vi "EnFlo_Lab_Temp_Control.vi"(0 "Current Time":dbl) -> ()   [LabVIEW 2022 SP3]
uses:
  Anemometry/Anemometry Sub Vis/Globals/EnFlo_Tunnel_Global.vi
  <vilib>/Analysis/NI_AALPro.lvlib
panel:
  in  "Don't Use Fan Heaters":bool
  in  "Don't Use Exit Heaters":bool
  out "At Maximum Heating":bool
  out "At Maximum Cooling":bool
  out "Back End Chiller Cooling Max":bool
  out "Back End Chiller Heating Max":bool
  out "Exit Heaters Max":bool
  out "Fan Heater Max":bool
  out "Volcano Max":bool
  out "Vent Max":bool
  out "Back End Chiller Cooling (kW)":dbl
  out "Ventilation Cooling (kW)":dbl
  out "Volcano Cooling (kW)":dbl
  out "Heat input to lab from Hot Pipework (kW)":dbl
  out "EnFlo_Lab Shut Down":bool
  in  "Paint Spraying by South West Fan":bool
  in  "Lab Fan heaters in kW":dbl=3.0
  in  "Don't Use Volcano":bool
  in  "Don't Use Ventilation":bool
  in  "Volcano Cooling kW":dbl=15.0
  in  "Manual Ventilation %":dbl=50.0
  in  "Lab Ventilation % during Ozone Exp":dbl
  in  "Ozone Averaging time (mins)":dbl=2.0
  in  "O3 Generator Control":T1={"Gen Output 0, Imin (mA)"=4.0, "USB3102 Number"=0.0, "DO O3 Gen Power"=0, "AO O3 Gen"=0, "O3 Gen Limit, Imax (mA)"=10.0, "Smoothing factor 0<1"=0.14} {"Smoothing factor 0<1" min=0.0 max=1.0 step=0.01; "AO O3 Gen" min=0 max=2 step=1; "DO O3 Gen Power" min=0 max=7 step=1}
  out "Ventilation Cooling limit in kW":dbl
  in  "Kp Ventilation":dbl=1.8
  out "Lab Reference Temperature":dbl
  out "Derivative Short":dbl(graph)
  in  "Kd Long":dbl=6000.0 format="%.2f"
  in  "Derivative Short History":i32=9
  in  "Exit Heater Power in kW":dbl=12.0
  out "Error":dbl(graph)
  out "Derivative Long":dbl(graph)
  out "integral":dbl(graph)
  out "Proportional":dbl(graph)
  out "Integral Term":dbl
  out "Derivative Term":dbl
  out "Proportional Term":dbl
  out "Cooling from Tunnel Exit Duct kW":dbl
  out "Exit Heater Dem Power %":dbl
  in  "Ki":dbl=0.013 format="%.3f"
  in  "Kp":dbl=3.0 format="%.2f"
  in  "Kd short":dbl=500.0 format="%.2f"
  in  "Derivative Long History":i32=35
  out "EnFlo Lab:labstrat1:Av Temp":dbl
  out "EnFlo_Tunnel:Exit Duct:Dem Temp":dbl
  out "Reduction in air temp from ambient":dbl
  out "Heat Extraction Value in kW":dbl
  out "EnFlo Lab:Desired:Air Temp":dbl
  out "Temperature Error":dbl
  # "USB 3102 Channel Numbers"
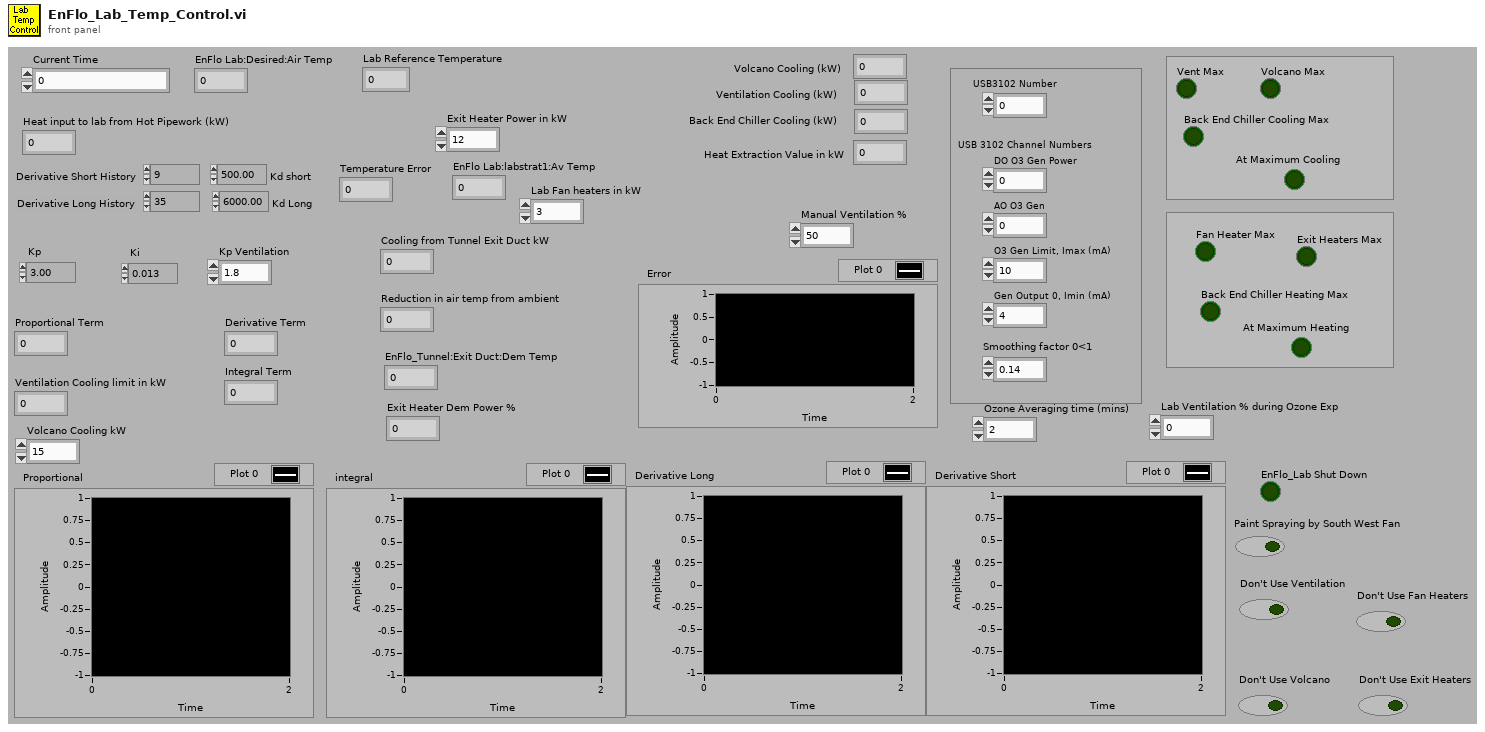
[diagram p1: front panel]
types:
  T1 = cluster{"Gen Output 0, Imin (mA)":sgl, "USB3102 Number":dbl, "DO O3 Gen Power":i32, "AO O3 Gen":i16, "O3 Gen Limit, Imax (mA)":dbl, "Smoothing factor 0<1":dbl}
  T2 = cluster{"second":i32, "minute":i32, "hour":i32, "day of month":i32, "month":i32, "year":i32, "day of week":i32, "day of year":i32, "is DST":i32}
  T3 = enum16{"Append to Global", "Read Global then Clear"}
  T4 = typedef "Ch_description_ADAM.ctl" = cluster{"Ch Name":string, "Type":T5, "Function":T6, "Ch State":T7, "Calibration type":T8, "A":dbl, "B":dbl, "C":dbl, "D":dbl, "Comments":string, "Address":T9, "String":string, "Duty":u16}
  T5 = typedef "Module_type_ADAM.ctl" = string
  T6 = typedef "Function_ADAM.ctl" = enum16{"Analogue Input", "Digital Input", "Event counter", "Event rate", "Analogue Output", "Digital Output", "Relay Output"}
  T7 = typedef "Channel_State.ctl" = enum16{"On", "Off", "Always On", "Always Off"}
  T8 = typedef "Calib_type_ADAM.ctl" = string
  T9 = typedef "Address.ctl" = cluster{"Main":i32, "Ch.":i32, "Sub":i32, "Port Name":string}
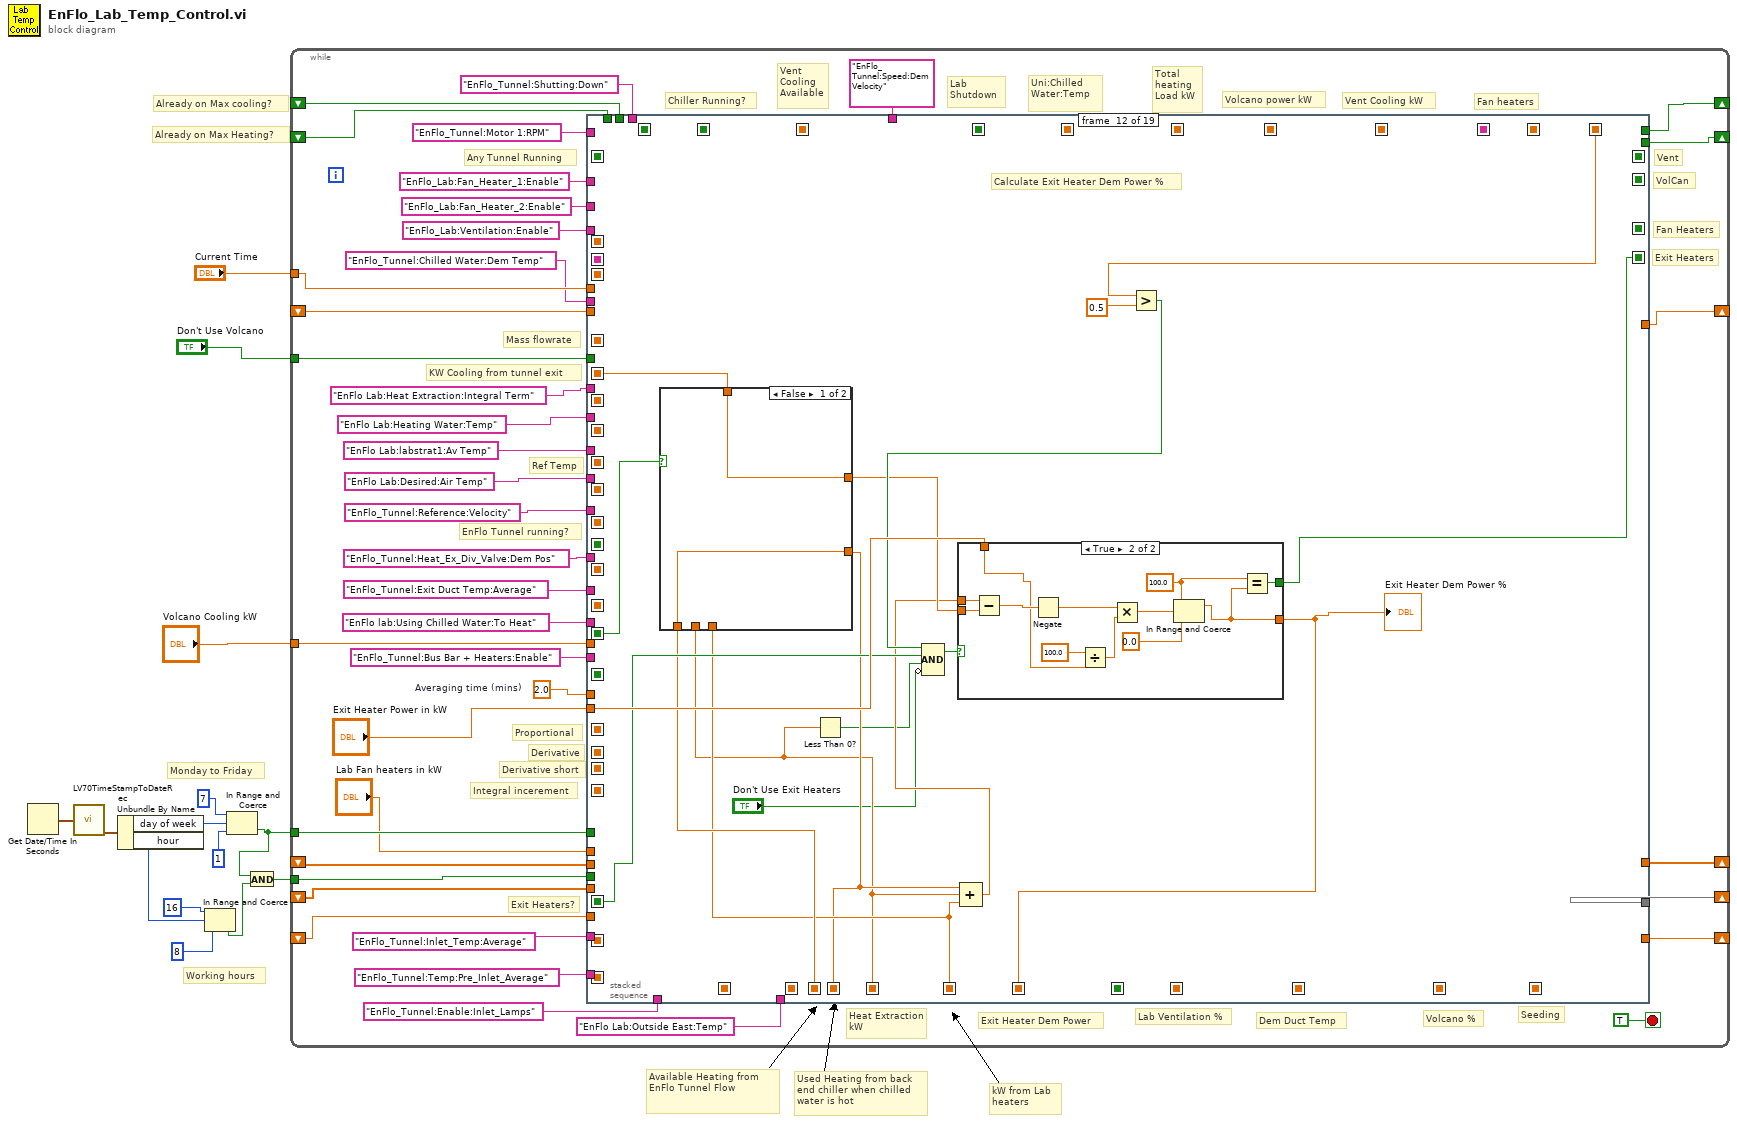
[diagram p0: block diagram]
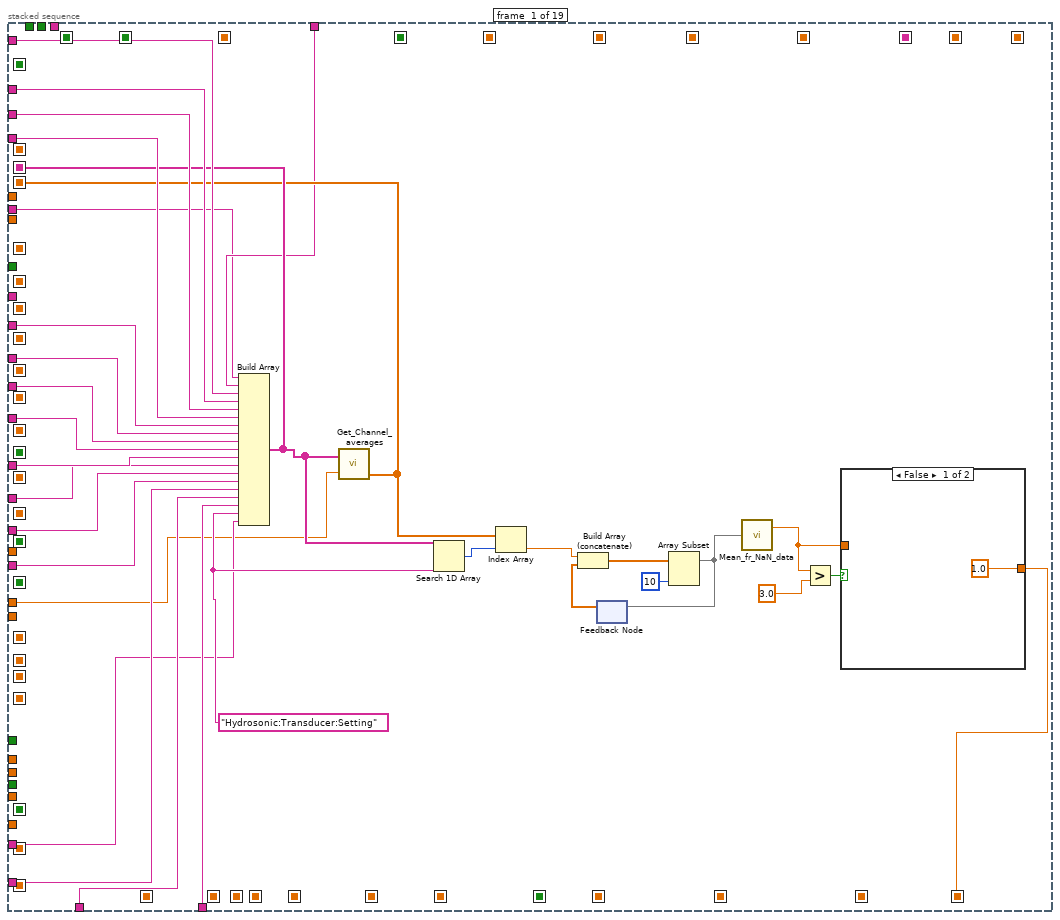
[diagram p2: hidden frame]
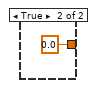
[diagram p3: hidden frame]
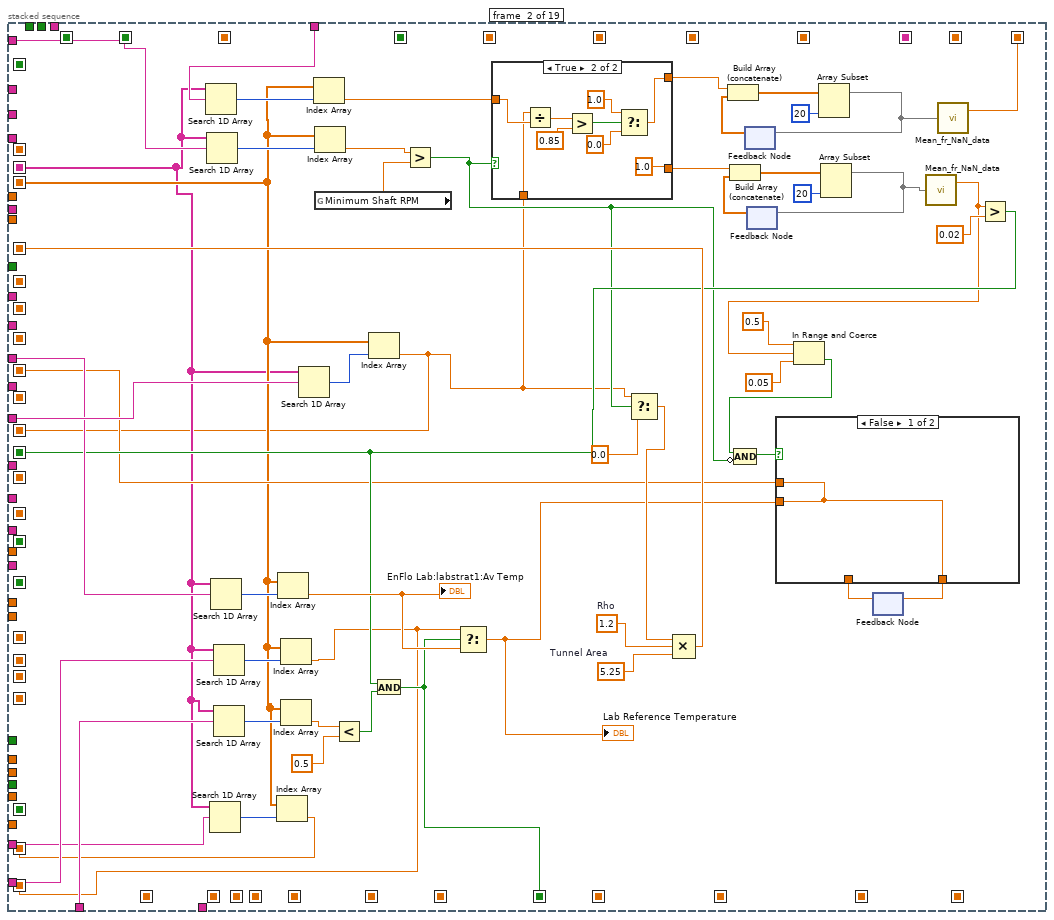
[diagram p4: hidden frame]
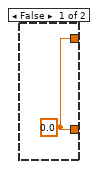
[diagram p5: hidden frame]
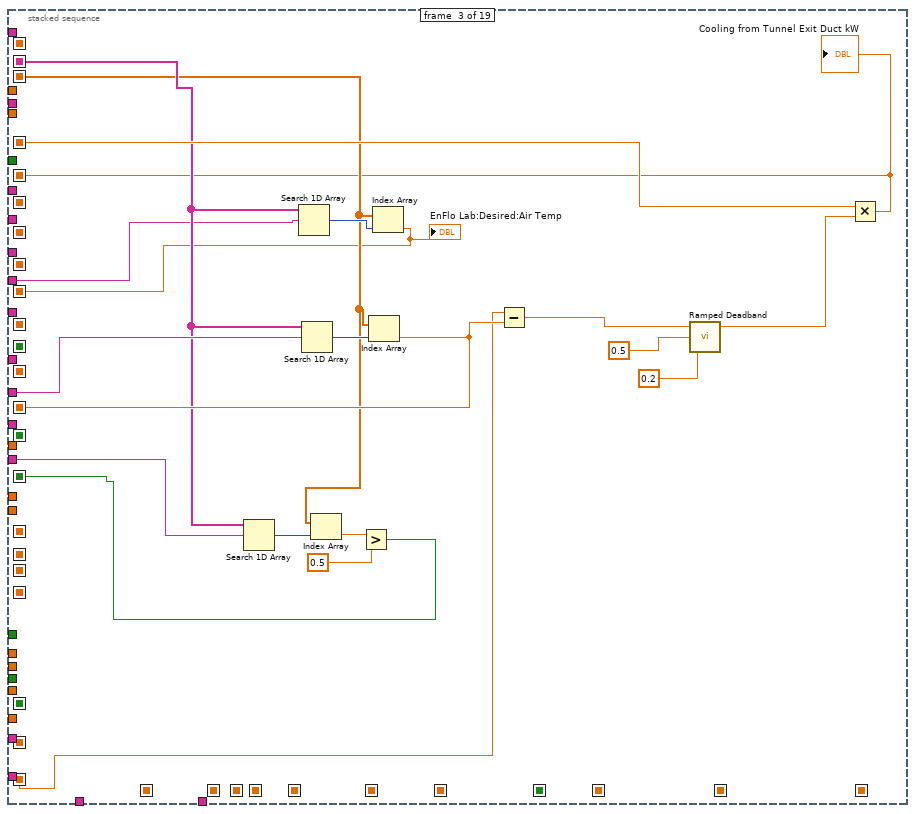
[diagram p7: hidden frame]
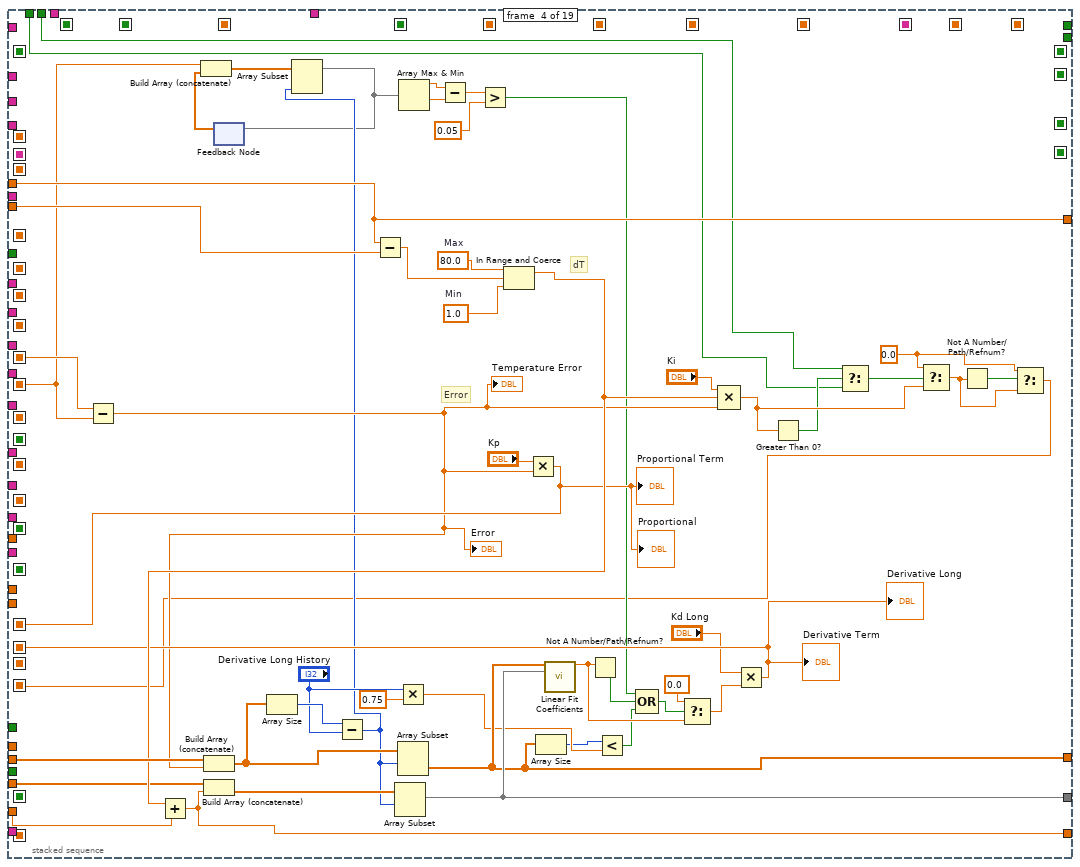
[diagram p8: hidden frame]
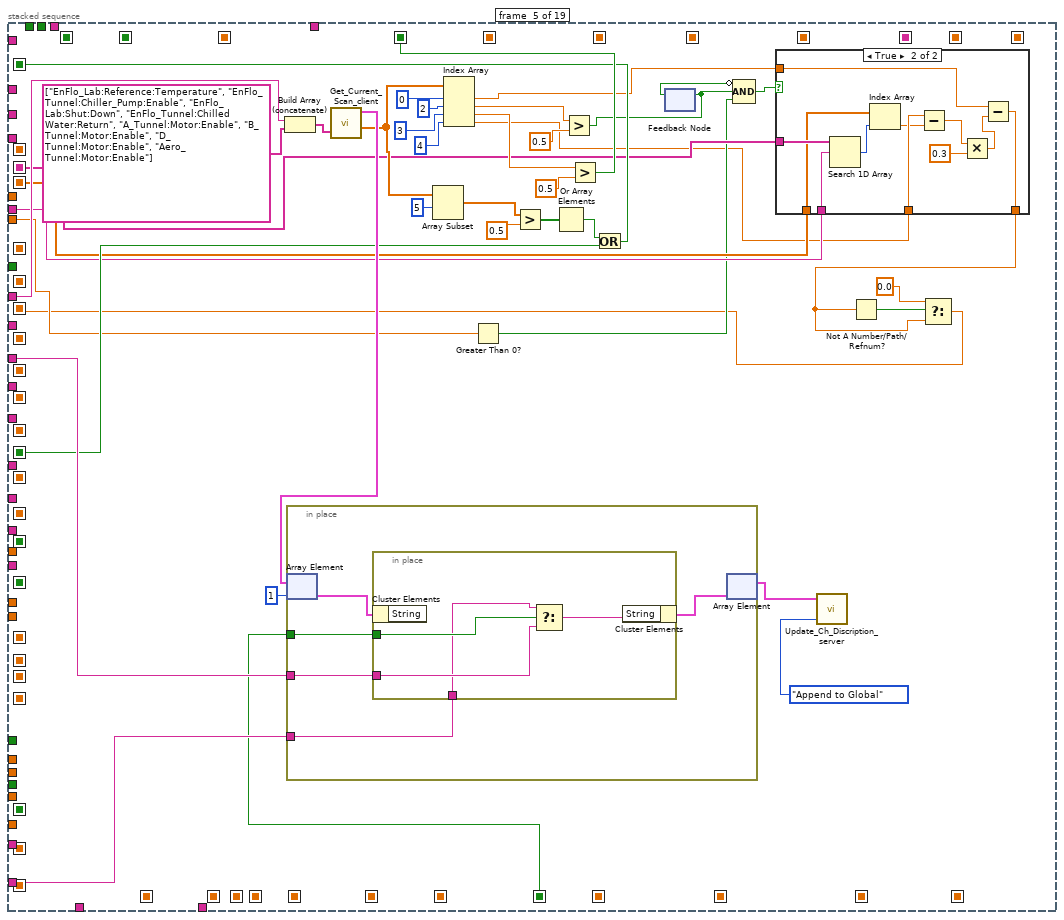
[diagram p9: hidden frame]
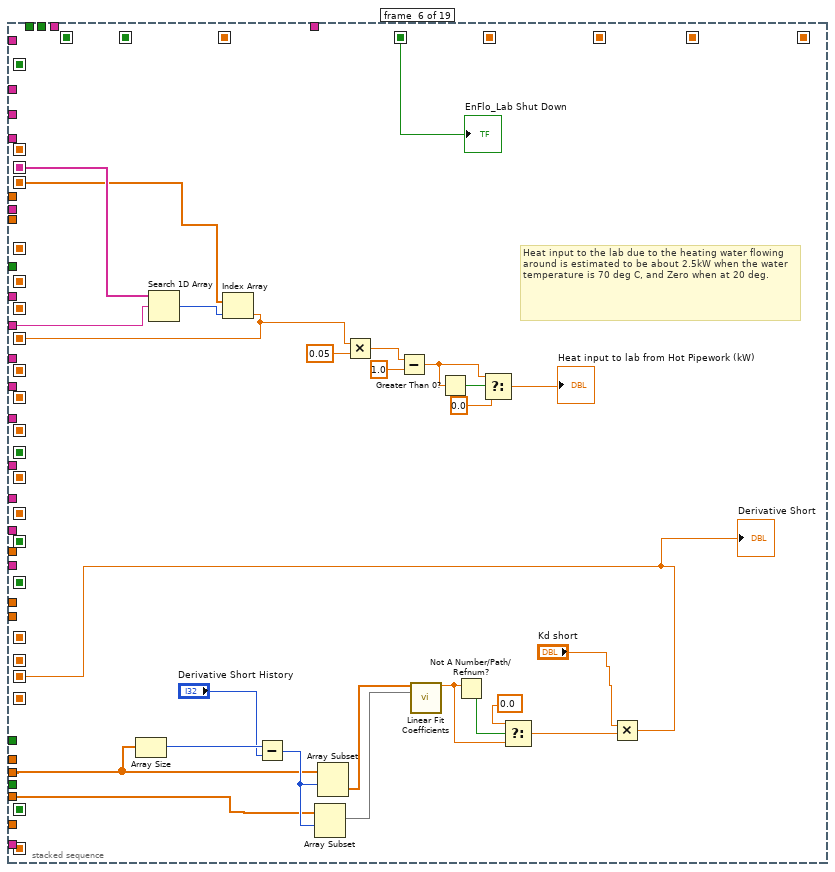
[diagram p11: hidden frame]
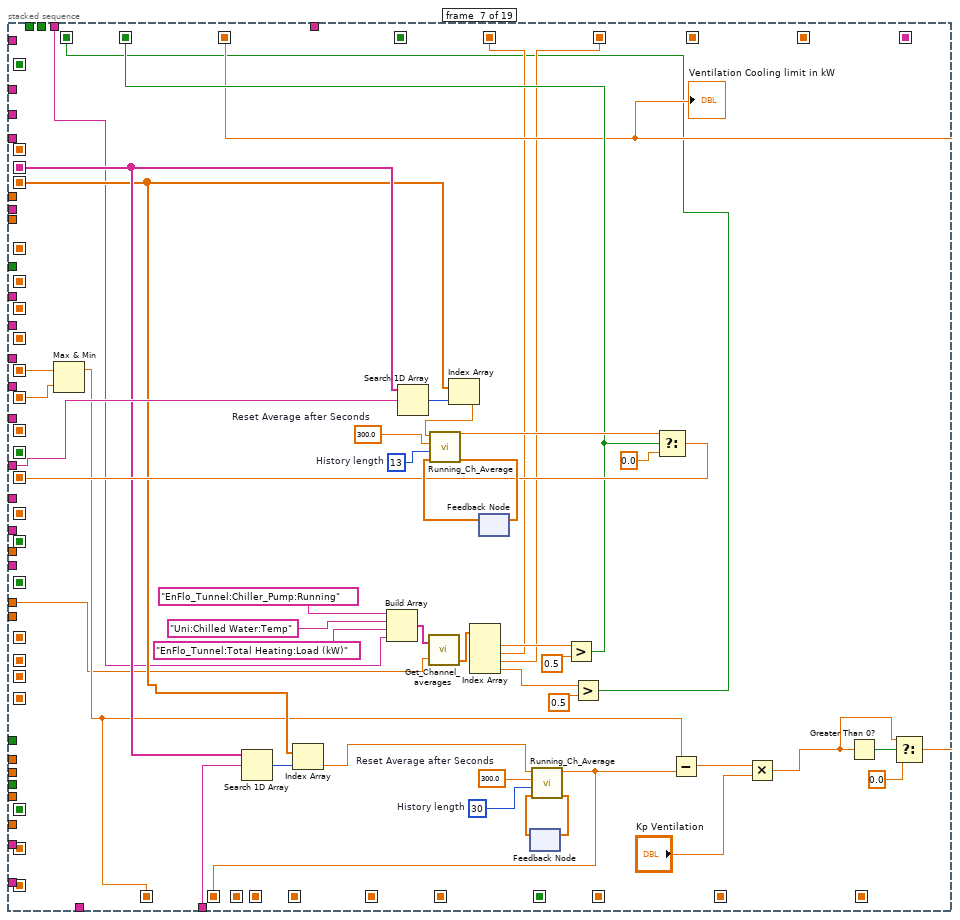
[diagram p12: hidden frame]
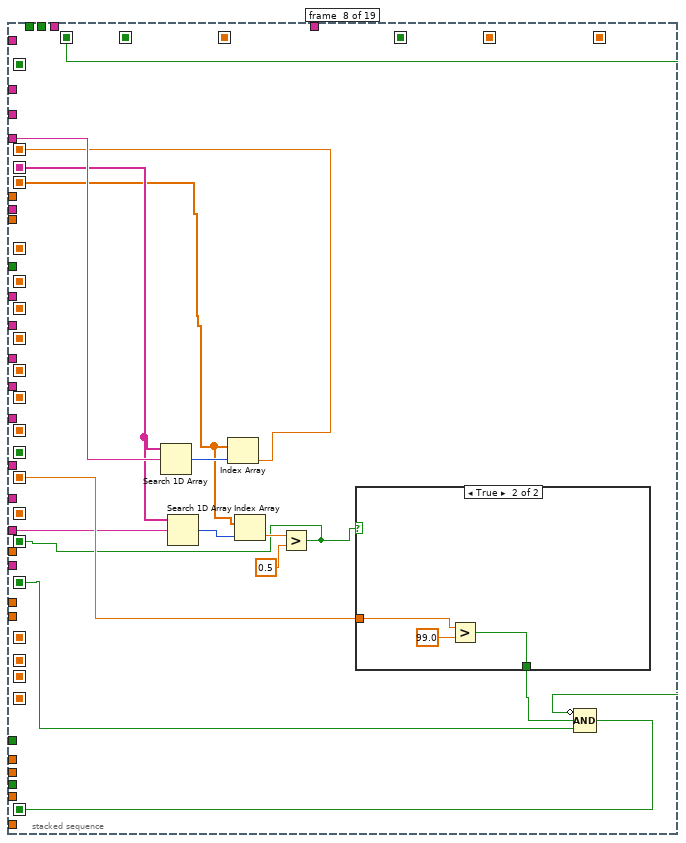
[diagram p13: hidden frame]
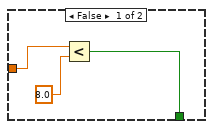
[diagram p14: hidden frame]
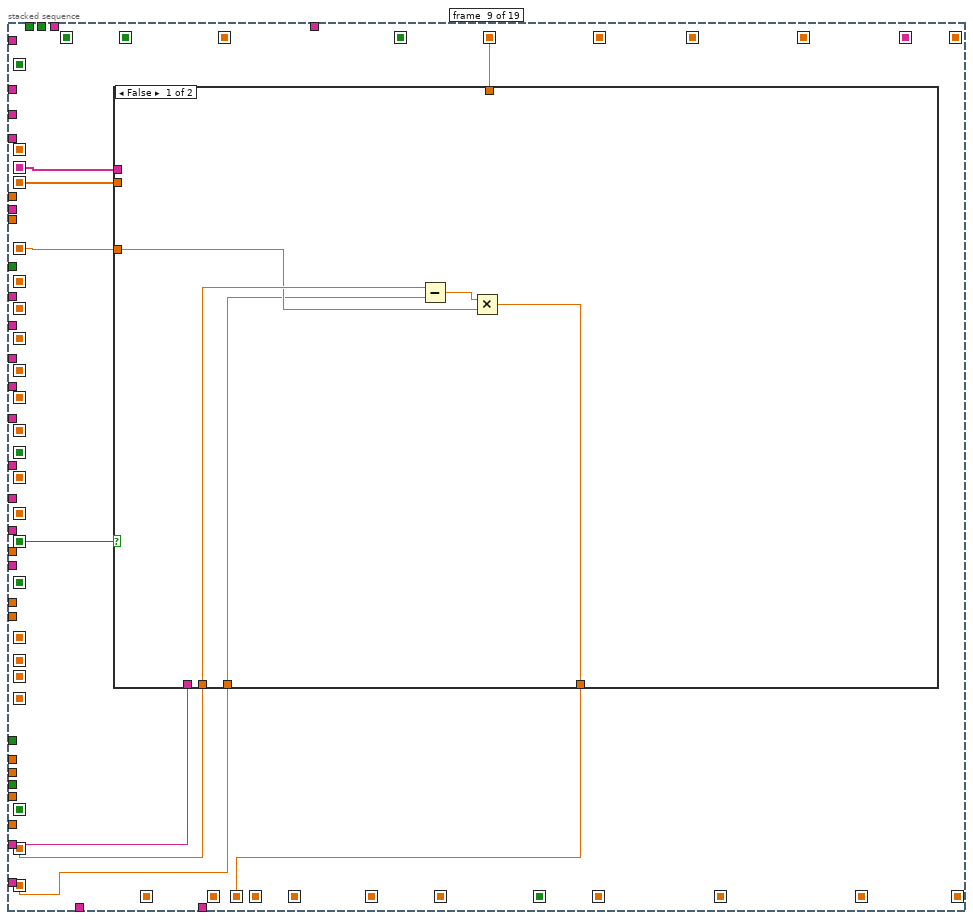
[diagram p15: hidden frame]
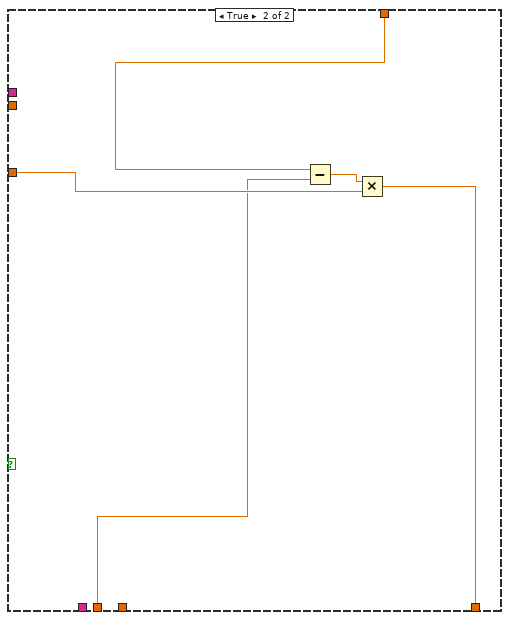
[diagram p16: hidden frame]
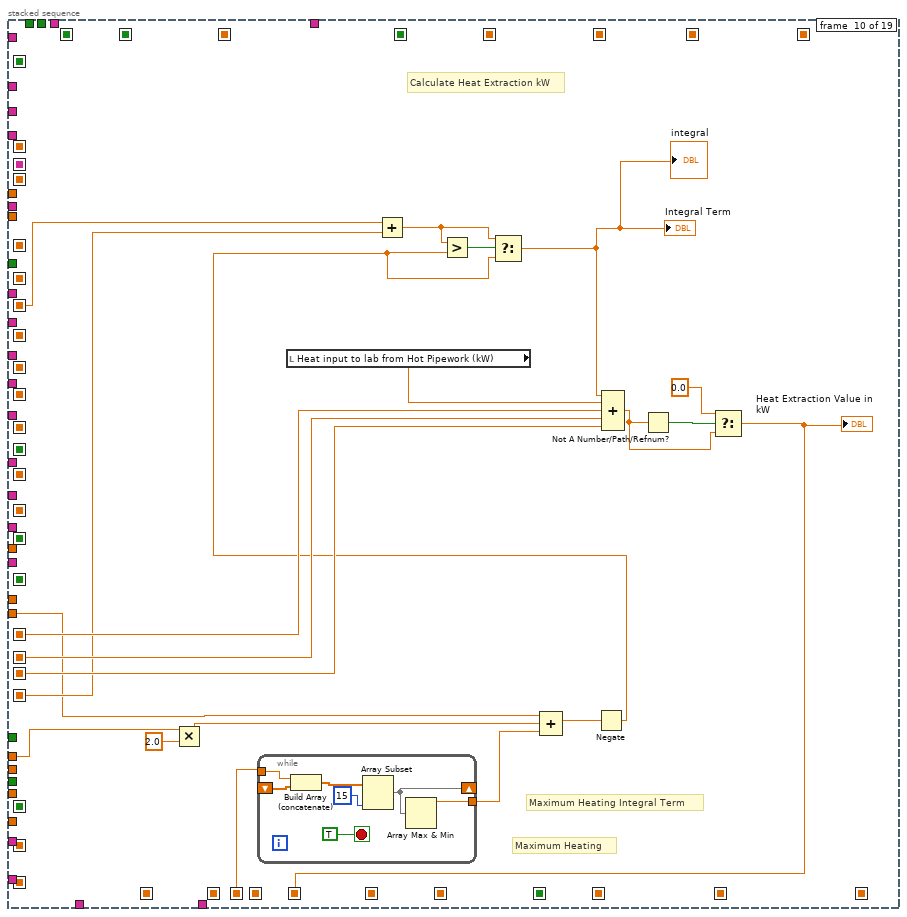
[diagram p17: hidden frame]
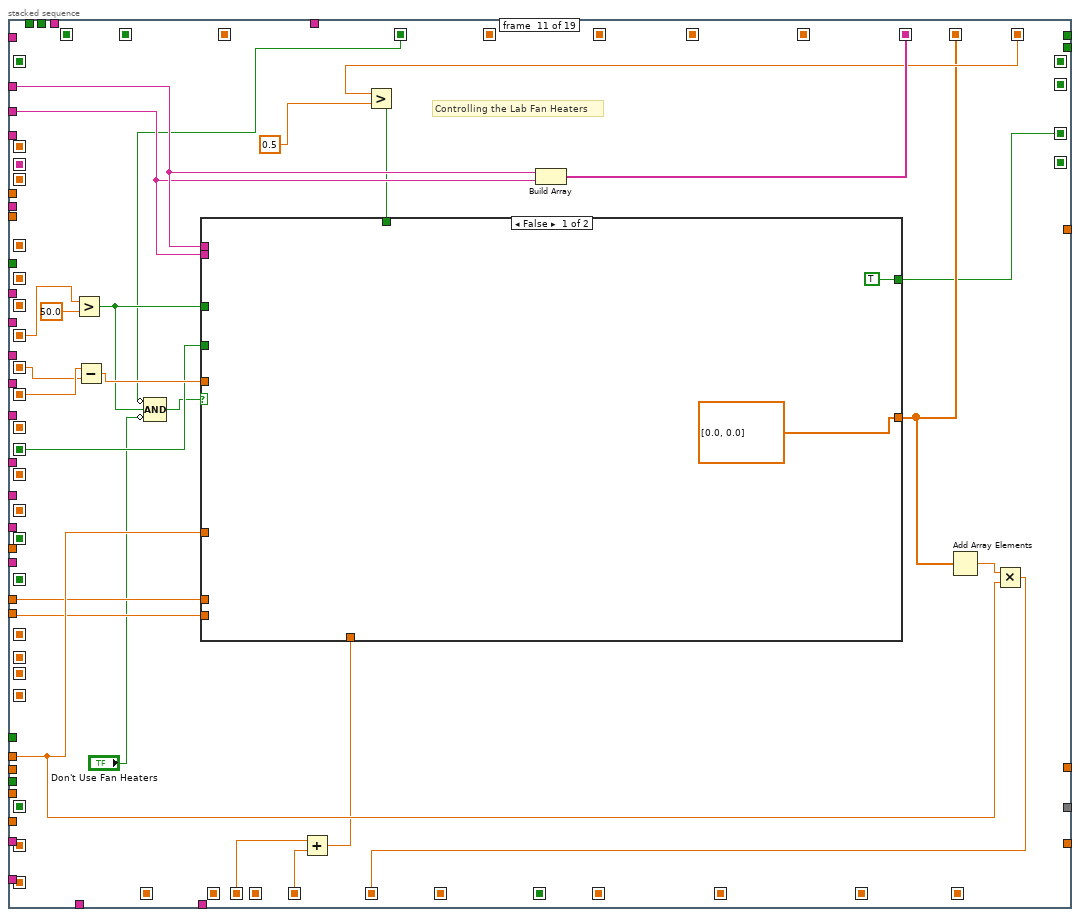
[diagram p18: hidden frame]
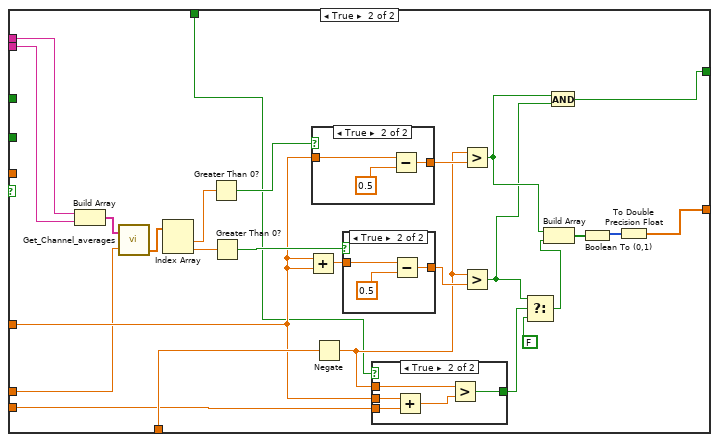
[diagram p19: hidden frame]
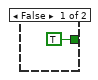
[diagram p20: hidden frame]
diagram:
  # "Already on Max Heating?"
  # "Already on Max cooling?"
  # "Used Heating from back end chiller when chilled water is hot"
  # "kW from Lab\nheaters"
  # "Available Heating from EnFlo Tunnel Flow"
  # "Monday to Friday"
  # "Working hours"
  n1 = Get Date/Time In Seconds() -> (seconds since 1Jan1904=w11:timestamp)
  n2 = call <vilib>:"LV70TimeStampToDateRec.vi"("time stamp"=w11) -> ("date time rec"=w13:T2)
  n3 = Unbundle By Name(w13) -> ("day of week"=w10:i32, "hour"=w6:i32)
  n4 = In Range and Coerce(upper limit=16, x=w6, lower limit=8) -> (In Range?=w3:bool)  [unwired: 1 out]
  n5 = In Range and Coerce(upper limit=7, x=w10, lower limit=1) -> (In Range?=w2:bool)  [unwired: 1 out]
  n6 = And(x=w2, y=w3) -> (x .and. y?=w1:bool)
  n7 = while {
    shift-right: [w44] -> _
    shift-left: _ -> [w45]
    shift-right: [w50] -> _
    shift-left: _ -> [w48]
    tunnel: "Current Time" -> [w49]
    shift-right: [w46] -> _
    shift-left: _ -> [w42]
    shift-right: [w47] -> _
    shift-left: _ -> [w43]
    tunnel: w2 -> [w29]
    tunnel: "Volcano Cooling kW" -> [w28]
    tunnel: "Don't Use Volcano" -> [w27]
    tunnel: w1 -> [w24]
    shift-right: [w19] -> _
    shift-left: _ -> [w18]
    shift-right: [w17] -> _
    shift-left: _ -> [w16]
    stop <- TRUE stop-if-true
    w21 = 2.0  # Averaging time (mins)
    # "Derivative short"
    # "Exit Heaters"
    # "Fan Heaters"
    # "VolCan"
    # "Vent"
    # "Any Tunnel Running"
    # "Lab\nShutdown"
    # "Total\nheating\nLoad kW"
    # "Seeding"
    # "Fan heaters"
    # "Dem Duct Temp"
    # "Volcano %"
    # "Chiller Running?"
    # "Volcano power kW"
    # "Uni:Chilled Water:Temp"
    # "Vent Cooling kW"
    # "Lab Ventilation %"
    # "Exit Heaters?"
    # "Exit Heater Dem Power"
    # "Heat Extraction kW"
    # "Vent Cooling Available"
    # "Ref Temp"
    # "EnFlo Tunnel running?"
    # "KW Cooling from tunnel exit"
    # "Mass flowrate"
    # "Integral incerement"
    # "Derivative"
    # "Proportional"
    n8 = stacked-sequence {
      seq-local: [w69 _ _ _ _ _ _ _ _ _ _ _ _ _ _ _ _ _ _] -> [_ w100 w165 _ w237 w300 w344 w360 w385 _ _ _ w552 _ _ _ _ w849 _]
      seq-local: [w71 _ _ _ _ _ _ _ _ _ _ _ _ _ _ _ _ _ _] -> [_ w99 w166 _ w238 w301 w345 w361 w384 _ _ _ w553 _ _ _ _ w851 _]
      seq-local: [_ _ _ w208 _ _ _ _ _ _ _ _ _ _ _ _ _ _ _] -> [_ _ _ _ _ _ _ _ _ w420 _ _ _ _ _ _ _ _ _]
      seq-local: [_ _ _ w207 _ _ _ _ _ _ _ _ _ _ _ _ _ _ _] -> [_ _ _ _ _ _ _ _ _ w419 _ _ _ _ _ _ _ _ _]
      seq-local: [_ _ _ w178 _ _ _ _ _ _ _ _ _ _ _ _ _ _ _] -> [_ _ _ _ _ _ _ _ _ w413 _ _ _ _ _ _ _ _ _]
      seq-local: [_ w140 _ _ _ _ _ _ _ _ _ _ _ _ _ _ _ _ _] -> [_ _ w175 _ _ _ _ _ w387 _ _ _ _ _ _ w758 _ _ _]
      seq-local: [_ _ w162 _ _ _ _ _ _ _ _ _ _ _ _ _ _ _ _] -> [_ _ _ _ _ _ _ _ _ _ _ w504 _ _ _ _ w815 _ _]
      seq-local: [_ _ w163 _ _ _ _ _ _ _ _ _ _ _ _ _ _ _ _] -> [_ _ _ w193 _ _ w334 _ _ _ w451 _ w556 _ _ w761 _ w847 _]
      seq-local: [_ _ w170 _ _ _ _ _ _ _ _ _ _ _ _ _ _ _ _] -> [_ _ _ _ _ _ _ w370 _ _ _ _ _ _ _ _ _ _ _]
      seq-local: [_ _ _ _ _ _ w348 _ _ _ _ _ _ _ _ _ _ _ _] -> [_ _ _ _ _ _ _ w368 _ _ _ _ _ _ w696 _ w819 w846 w875]
      seq-local: [_ w113 _ _ _ _ _ _ _ _ _ _ _ _ _ _ _ _ _] -> [_ _ _ w205 _ _ w335 _ _ _ w450 _ w551 _ w702 w769 _ _ _]
      seq-local: [_ _ w168 _ _ _ _ _ _ _ _ _ _ _ _ _ _ _ _] -> [_ _ _ _ _ _ _ _ _ _ _ _ _ _ _ _ _ _ _]
      seq-local: [_ _ _ _ _ w303 _ _ _ _ _ _ _ _ _ _ _ _ _] -> [_ _ _ _ _ _ _ _ _ w416 _ _ _ _ _ _ _ _ _]
      seq-local: [_ w118 _ _ _ _ _ _ _ _ _ _ _ _ _ _ _ _ _] -> [_ _ _ _ w254 _ _ _ _ _ w445 _ _ _ _ _ _ w839 w874]
      seq-local: [_ _ _ _ _ _ _ w372 _ _ _ _ _ _ _ _ _ _ _] -> [_ _ _ _ _ _ _ _ _ _ _ _ w545 _ _ _ _ _ _]
      seq-local: [_ _ _ _ _ w295 _ _ _ _ _ _ _ _ _ _ _ _ _] -> [_ _ _ _ _ _ _ _ _ _ w452 _ w547 _ _ _ _ _ _]
      seq-local: [_ _ _ _ _ _ w329 _ _ _ _ _ _ _ _ _ _ _ _] -> [_ _ _ _ _ _ _ _ _ _ _ _ w550 w629 _ _ w830 _ _]
      seq-local: [_ _ _ _ _ _ _ _ _ w415 _ _ _ _ _ _ _ _ _] -> [_ _ _ _ _ _ _ _ _ _ w438 w498 w549 _ w699 w772 w827 _ _]
      seq-local: [_ _ _ _ _ _ _ _ _ _ _ w507 _ _ _ _ _ _ _] -> [_ _ _ _ _ _ _ _ _ _ _ _ w548 _ _ _ w828 _ _]
      seq-local: [_ _ _ _ _ _ _ _ _ _ _ _ w546 _ _ _ _ _ _] -> [_ _ _ _ _ _ _ _ _ _ _ _ _ w630 _ _ _ _ _]
      seq-local: [_ w123 _ _ _ _ _ _ _ _ _ _ _ _ _ _ _ _ _] -> [_ _ _ _ w262 _ _ _ _ _ _ _ _ _ _ _ _ _ _]
      seq-local: [_ _ _ _ _ _ _ w369 _ _ _ _ _ _ _ _ _ _ _] -> [_ _ _ _ _ _ _ _ _ _ _ w510 _ _ _ _ _ _ _]
      seq-local: [_ _ _ _ _ _ w333 _ _ _ _ _ _ _ _ _ _ _ _] -> [_ _ _ _ _ _ _ _ _ _ _ _ w544 _ _ _ _ _ _]
      seq-local: [_ _ _ _ _ _ _ _ _ _ _ _ _ w617 _ _ _ _ _] -> [_ _ _ _ _ _ _ _ _ _ _ _ _ _ w700 w774 w829 _ _]
      seq-local: [_ _ _ _ _ _ w326 _ _ _ _ _ _ _ _ _ _ _ _] -> [_ _ _ _ _ _ _ _ w388 _ _ _ w543 _ w701 _ _ w848 _]
      seq-local: [_ _ _ _ _ _ _ _ _ _ _ _ _ _ w695 _ _ _ _] -> [_ _ _ _ _ _ _ _ _ _ _ _ _ _ _ w773 w821 _ _]
      seq-local: [_ _ _ _ _ _ w332 _ _ _ _ _ _ _ _ _ _ _ _] -> [_ _ _ _ _ _ _ _ _ _ _ _ _ _ w698 w757 _ w836 _]
      seq-local: [_ _ _ _ _ _ w325 _ _ _ _ _ _ _ _ _ _ _ _] -> [_ _ _ _ _ _ _ _ _ _ _ _ w541 _ _ _ _ _ _]
      seq-local: [_ _ _ _ _ _ _ _ _ _ _ _ _ _ w689 _ _ _ _] -> [_ _ _ _ _ _ _ _ _ _ _ _ _ _ _ w755 w826 _ _]
      seq-local: [_ _ _ _ _ _ _ _ _ _ _ _ _ _ _ w767 _ _ _] -> [_ _ _ _ _ _ _ _ _ _ _ _ _ _ _ _ w825 _ _]
      seq-local: [_ _ _ _ _ _ _ _ _ _ w448 _ _ _ _ _ _ _ _] -> [_ _ _ _ _ _ _ _ _ _ _ _ _ _ _ _ w823 _ _]
      seq-local: [_ _ _ _ _ _ _ _ _ _ w435 _ _ _ _ _ _ _ _] -> [_ _ _ _ _ _ _ _ _ _ _ _ _ _ _ _ w824 _ _]
      seq-local: [_ w93 _ _ _ _ _ _ _ _ _ _ _ _ _ _ _ _ _] -> [_ _ _ _ _ _ _ _ _ _ w441 w512 _ _ _ _ _ _ _]
      seq-local: [w58 _ _ _ _ _ _ _ _ _ _ _ _ _ _ _ _ _ _] -> [_ _ _ _ _ _ _ _ _ _ _ _ w540 _ _ _ _ _ _]
      seq-local: [_ _ _ _ _ _ w323 _ _ _ _ _ _ _ _ _ _ _ _] -> [_ _ _ _ _ _ _ _ _ _ _ _ _ _ _ _ w816 _ _]
      seq-local: [_ _ _ _ _ _ w319 _ _ _ _ _ _ _ _ _ _ _ _] -> [_ _ _ _ _ _ _ w363 _ _ _ _ _ _ _ _ _ _ _]
      seq-local: [_ _ _ _ w260 _ _ _ _ _ _ _ _ _ _ _ _ _ _] -> [_ _ _ _ _ w290 _ _ _ _ w439 _ _ w618 w693 _ _ _ _]
      seq-local: [_ _ _ _ w253 _ _ _ _ _ _ _ _ _ _ _ _ _ _] -> [_ _ _ _ _ _ _ _ _ _ _ _ _ _ w690 _ _ _ _]
      seq-local: [_ _ _ _ _ _ _ w362 _ _ _ _ _ _ _ _ _ _ _] -> [_ _ _ _ _ _ _ _ w389 _ _ w506 _ _ _ w765 _ w837 w873]
      seq-local: [_ _ _ _ _ _ _ _ w386 _ _ _ _ _ _ _ _ _ _] -> [_ _ _ _ _ _ _ _ _ w406 w437 w502 _ _ _ w764 _ _ _]
      seq-local: [_ _ _ _ _ _ _ _ _ _ w434 _ _ _ _ _ _ _ _] -> [_ _ _ _ _ _ _ _ _ _ _ w501 _ _ _ w763 _ _ _]
      seq-local: [_ _ _ _ _ _ _ _ _ _ _ w500 _ _ _ _ _ _ _] -> [_ _ _ _ _ _ _ _ _ _ _ _ _ _ _ w762 _ _ _]
      seq-local: [_ w97 _ _ _ _ _ _ _ _ _ _ _ _ _ _ _ _ _] -> [_ _ _ _ _ _ _ _ w382 _ _ _ _ _ _ _ _ _ _]
      seq-local: [_ w96 _ _ _ _ _ _ _ _ _ _ _ _ _ _ _ _ _] -> [_ _ w161 _ _ _ _ _ w381 _ _ _ _ _ _ _ _ _ _]
      seq-local: [_ _ _ _ _ _ _ _ _ _ _ _ w537 _ _ _ _ _ _] -> [_ _ _ _ _ _ _ _ _ _ _ _ _ _ _ _ _ w845 w871]
      seq-local: [_ _ _ _ _ _ _ _ _ _ _ _ _ _ w688 _ _ _ _] -> [_ _ _ _ _ _ _ _ _ _ _ _ _ _ _ _ _ w844 w870]
      seq-local: [_ _ _ _ _ _ _ _ _ _ w429 _ _ _ _ _ _ _ _] -> [_ _ _ _ _ _ _ _ _ _ _ _ _ _ _ _ _ _ w876]
      seq-local: [_ _ _ _ _ _ _ _ _ _ _ w499 _ _ _ _ _ _ _] -> [_ _ _ _ _ _ _ _ _ _ _ _ _ _ _ _ _ _ w877]
      seq-local: [_ _ _ _ w228 _ _ _ _ _ _ _ _ _ _ _ _ _ _] -> [_ _ _ _ _ _ _ _ _ w412 _ _ _ _ _ _ _ w840 w866]
      seq-local: [_ w90 _ _ _ _ _ _ _ _ _ _ _ _ _ _ _ _ _] -> [_ _ _ _ _ _ _ _ _ _ _ _ _ _ _ _ _ _ _]
      tunnel: "EnFlo Lab:labstrat1:Av Temp" -> [w87 w128 _ _ w268 _ _ _ _ _ _ _ _ _ _ _ _ _ _]
      tunnel: "EnFlo Lab:Desired:Air Temp" -> [w86 _ w164 _ _ _ _ _ _ _ _ _ _ _ _ _ _ _ _]
      tunnel: "EnFlo_Tunnel:Reference:Velocity" -> [w85 w141 _ _ _ _ _ _ _ _ _ _ _ _ _ _ _ _ _]
      tunnel: "EnFlo_Tunnel:Heat_Ex_Div_Valve:Dem Pos" -> [w84 _ _ _ _ _ w355 _ _ _ _ _ _ _ _ _ _ _ _]
      tunnel: "EnFlo_Tunnel:Exit Duct Temp:Average" -> [w83 _ w176 _ _ _ _ _ _ _ _ _ _ _ _ _ _ _ _]
      tunnel: [_ _ _ w227 _ _ _ _ _ _ _ _ _ _ _ _ _ _ _] -> w50
      tunnel: w49 -> [_ _ _ w227 _ _ _ _ _ _ _ _ _ _ _ _ _ _ _]
      tunnel: w48 -> [_ _ _ w226 w235 _ _ _ _ _ _ _ _ _ _ _ _ _ _]
      tunnel: [_ _ _ w204 _ _ _ _ _ _ _ _ _ _ _ _ _ _ _] -> w47
      tunnel: [_ _ _ w217 _ _ _ _ _ _ _ _ _ _ _ _ _ _ _] -> w46
      tunnel: w45 -> [_ _ _ w216 _ _ _ _ _ _ _ _ _ _ _ _ _ _ _]
      tunnel: [_ _ _ w215 _ _ _ _ _ _ _ _ _ _ _ _ _ _ _] -> w44
      tunnel: w43 -> [_ _ _ w214 _ w308 _ _ _ _ _ _ _ _ _ _ _ _ _]
      tunnel: w42 -> [_ _ _ w209 _ w309 _ _ _ _ _ _ _ _ _ _ _ _ _]
      tunnel: "EnFlo_Tunnel:Bus Bar + Heaters:Enable" -> [w78 _ w171 _ _ _ _ _ _ _ _ _ _ _ _ _ _ _ _]
      tunnel: "Exit Heater Power in kW" -> [_ _ _ _ _ _ _ _ _ w407 w431 w513 _ _ _ _ _ _ _]
      tunnel: "EnFlo_Lab:Fan_Heater_1:Enable" -> [w82 _ _ _ _ _ _ _ _ _ w449 _ _ _ _ _ _ _ _]
      tunnel: "EnFlo_Lab:Fan_Heater_2:Enable" -> [w81 _ _ _ _ _ _ _ _ _ w446 _ _ _ _ _ _ _ _]
      tunnel: "EnFlo_Lab:Ventilation:Enable" -> [w80 _ _ _ _ _ _ w373 _ _ _ _ _ _ _ _ _ _ _]
      tunnel: "EnFlo_Tunnel:Motor 1:RPM" -> [w79 w136 _ _ _ _ _ _ _ _ _ _ _ _ _ _ _ _ _]
      tunnel: "EnFlo Lab:Heating Water:Temp" -> [w77 _ _ _ _ w299 _ _ _ _ _ _ _ _ _ _ _ _ _]
      tunnel: "EnFlo_Tunnel:Temp:Pre_Inlet_Average" -> [w76 w129 _ _ w267 _ _ _ _ _ _ _ _ _ _ _ _ _ _]
      tunnel: "EnFlo_Tunnel:Enable:Inlet_Lamps" -> [w75 w130 _ _ _ _ _ _ _ _ _ _ _ _ _ _ _ _ _]
      tunnel: "EnFlo Lab:Outside East:Temp" -> [w74 _ _ _ _ _ w343 _ _ _ _ _ _ _ _ _ _ _ _]
      tunnel: "EnFlo lab:Using Chilled Water:To Heat" -> [w73 _ _ _ _ _ _ w366 _ _ _ _ _ _ _ _ _ _ _]
      tunnel: w29 -> [_ _ _ _ _ _ _ _ _ _ _ _ _ _ _ _ _ _ _]
      tunnel: w28 -> [_ _ _ _ _ _ _ _ _ _ _ _ _ _ w697 _ _ _ _]
      tunnel: w27 -> [_ _ _ _ _ _ _ _ _ _ _ _ w542 _ w687 w754 _ _ _]
      tunnel: "Lab Fan heaters in kW" -> [_ _ _ _ _ _ _ _ _ w410 w433 _ _ _ _ _ _ _ _]
      tunnel: "EnFlo_Tunnel:Shutting:Down" -> [_ _ _ _ _ _ w322 _ _ _ _ _ _ _ _ _ _ _ _]
      tunnel: w24 -> [_ _ _ _ _ _ _ _ _ _ _ _ w539 _ w691 _ _ _ _]
      tunnel: "EnFlo_Tunnel:Speed:Dem Velocity" -> [w64 w108 _ _ _ _ _ _ _ _ _ _ _ _ _ _ _ _ _]
      tunnel: "EnFlo_Tunnel:Inlet_Temp:Average" -> [w63 w98 _ _ _ _ _ _ w383 _ _ _ _ _ _ _ _ _ _]
      tunnel: w21 -> [w62 _ _ _ _ _ w316 _ _ _ w430 _ w538 w614 _ _ _ _ _]
      tunnel: "EnFlo_Tunnel:Chilled Water:Dem Temp" -> [w60 _ _ _ w236 _ _ _ _ _ _ _ _ _ _ _ _ w850 _]
      tunnel: [_ _ _ _ _ _ _ _ _ _ _ _ _ _ _ _ _ w843 _] -> w19
      tunnel: w18 -> [_ _ _ w183 _ _ _ _ _ _ _ _ _ _ _ _ _ _ _]
      tunnel: [_ _ _ _ _ _ _ _ _ _ _ _ _ _ _ _ _ _ w869] -> w17
      tunnel: w16 -> [_ _ _ w182 _ _ _ _ _ _ _ _ _ _ _ _ _ _ _]
      tunnel: "EnFlo Lab:Heat Extraction:Integral Term" -> [_ _ _ _ w251 _ _ _ _ _ _ _ _ _ _ _ w811 _ _]
      frame #0 {
        w72 = "Hydrosonic:Transducer:Setting"
        n9 = Build Array(w60, w64, w79, w82, w81, w80, w77, w87, w86, w85, w84, w83, w73, w78, w76, w75, w74, w72, w63) -> (w71:string[])
        n10 = call "Get_Channel_averages.vi"("Desired Ch Names"=w71, "Averaging time (mins)"=w62) -> ("number"=w69:dbl[])  [unwired: 1 in, 2 out]
        n11 = Search 1D Array(1D array=w71, element=w72) -> (index of element=w70:i32)  [unwired: 1 out]
        n12 = Index Array(array=w69, index=w70) -> (element=w65:dbl)
        n13 = feedback #1() -> (w68:dbl[])  [unwired: 1 in]
        n14 = Build Array (concatenate)(w65, w68) -> (w66:dbl[])
        n15 = Array Subset(array=w66, length=10) -> (w61:dbl[])  [unwired: 1 in]
        n16 = feedback-in #1(w61) -> ()
        n17 = call "Mean_fr_NaN_data.vi"("Data"=w61) -> ("Mean value"=w56:dbl)  [unwired: 1 out]
        n18 = Greater?(x=w56, y=3.0) -> (0:w57:bool)
        n19 = case shown="False" w57 {
          tunnel: [1.0 ("f") 0.0 ("f")] -> w58
          tunnel: w56 -> [_ _]
          frame False {
          }
          frame True {
          }
        }
      }
      frame #1 {
        w144 = 5.25  # Tunnel Area
        w143 = 1.2  # Rho
        n20 = Search 1D Array(1D array=w99, element=w108) -> (index of element=w109:i32)  [unwired: 1 out]
        n21 = Search 1D Array(1D array=w99, element=w136) -> (index of element=w137:i32)  [unwired: 1 out]
        n22 = Search 1D Array(1D array=w99, element=w98) -> (index of element=w101:i32)  [unwired: 1 out]
        n23 = Search 1D Array(1D array=w99, element=w128) -> (index of element=w133:i32)  [unwired: 1 out]
        n24 = Search 1D Array(1D array=w99, element=w129) -> (index of element=w132:i32)  [unwired: 1 out]
        n25 = Search 1D Array(1D array=w99, element=w130) -> (index of element=w131:i32)  [unwired: 1 out]
        n26 = Index Array(array=w100, index=w101) -> (element=w97:dbl)
        n27 = Index Array(array=w100, index=w133) -> (element=w124:dbl)
        "EnFlo Lab:labstrat1:Av Temp" <- w124
        n28 = Index Array(array=w100, index=w132) -> (element=w96:dbl)
        n29 = Index Array(array=w100, index=w131) -> (element=w127:dbl)
        n30 = Search 1D Array(1D array=w99, element=w141) -> (index of element=w142:i32)  [unwired: 1 out]
        n31 = Index Array(array=w100, index=w109) -> (element=w106:dbl)
        n32 = Index Array(array=w100, index=w137) -> (element=w135:dbl)
        n33 = global read "EnFlo_Tunnel_Global.vi" "Minimum Shaft RPM"() -> (w134:dbl)
        n34 = Less?(x=w127, y=0.5) -> (x < y?=w125:bool)
        n35 = Index Array(array=w100, index=w142) -> (element=w90:dbl)
        n36 = Greater?(x=w135, y=w134) -> (0:w95:bool)
        n37 = case shown="True" w95 {
          tunnel: [w145 1.0 ("f")] -> w107
          tunnel: w106 -> [_ w150]
          tunnel: w90 -> [_ w149]
          tunnel: [w145 w147] -> w102
          frame False {
            w145 = 0.0 ("f")
          }
          frame True {
            n38 = Divide(x=w149, y=w150) -> (x/y=w146:dbl)
            n39 = Greater?(x=w146, y=0.85) -> (0:w151:bool)
            n40 = Select(t=1.0, s=w151, f=0.0) -> (s? t:f=w147:dbl)
          }
        }
        n41 = Select(t=w90, s=w95, f=0.0) -> (s? t:f=w138:dbl)
        n42 = Compound Arithmetic op=MULTIPLY(w138, w143, w144) -> (w140:dbl)
        n43 = feedback #2() -> (w104:dbl[])  [unwired: 1 in]
        n44 = Build Array (concatenate)(w102, w104) -> (w103:dbl[])
        n45 = feedback #3() -> (w121:dbl[])  [unwired: 1 in]
        n46 = Build Array (concatenate)(w107, w121) -> (w122:dbl[])
        n47 = Array Subset(array=w103, length=20) -> (w94:dbl[])  [unwired: 1 in]
        n48 = feedback-in #2(w94) -> ()
        n49 = Array Subset(array=w122, length=20) -> (w92:dbl[])  [unwired: 1 in]
        n50 = feedback-in #3(w92) -> ()
        n51 = feedback #4() -> (w112:dbl)  [unwired: 1 in]
        n52 = call "Mean_fr_NaN_data.vi"("Data"=w92) -> ("Mean value"=w91:dbl)  [unwired: 1 out]
        n53 = In Range and Coerce(upper limit=0.5, x=w91, lower limit=0.05) -> (In Range?=w111:bool)  [unwired: 1 out]
        n54 = Compound Arithmetic op=AND(w111, invert w95) -> (w110:bool)
        n55 = call "Mean_fr_NaN_data.vi"("Data"=w94) -> ("Mean value"=w93:dbl)  [unwired: 1 out]
        n56 = Greater?(x=w91, y=0.02) -> (0:w118:bool)
        n57 = And(x=w118, y=w125) -> (x .and. y?=w123:bool)
        n58 = Select(t=w96, s=w123, f=w124) -> (s? t:f=w114:dbl)
        "Lab Reference Temperature" <- w114
        n59 = case shown="False" w110 {
          tunnel: [w155 w156] -> w115
          tunnel: w114 -> [w155 _]
          tunnel: [w155 w156] -> w113
          tunnel: w112 -> [_ w156]
          frame False {
          }
          frame True {
          }
        }
        n60 = feedback-in #4(w115) -> ()
      }
      frame #2 {
        n61 = Search 1D Array(1D array=w166, element=w171) -> (index of element=w174:i32)  [unwired: 1 out]
        n62 = Search 1D Array(1D array=w166, element=w164) -> (index of element=w169:i32)  [unwired: 1 out]
        n63 = Search 1D Array(1D array=w166, element=w176) -> (index of element=w167:i32)  [unwired: 1 out]
        n64 = Index Array(array=w165, index=w174) -> (element=w173:dbl)
        n65 = Greater?(x=w173, y=0.5) -> (0:w170:bool)
        n66 = Index Array(array=w165, index=w167) -> (element=w168:dbl)
        n67 = Index Array(array=w165, index=w169) -> (element=w163:dbl)
        "EnFlo Lab:Desired:Air Temp" <- w163
        n68 = Subtract(x=w161, y=w168) -> (x-y=w159:dbl)
        n69 = call "Ramped Deadband.vi"("End of Ramp down"=0.2, "Beginning of Ramp Down"=0.5, "Error Value In"=w159) -> ("Error Value out"=w160:dbl)  [unwired: 2 in]
        n70 = Multiply(x=w175, y=w160) -> (x*y=w162:dbl)
        "Cooling from Tunnel Exit Duct kW" <- w162
      }
      frame #3 {
        w177 = 0.0 ("t")
        w225 = 1.0  # Min
        w224 = 80.0  # Max
        # "dT"
        # "Error"
        n71 = Subtract(x=w205, y=w193) -> (x-y=w196:dbl)
        "Temperature Error" <- w196
        "Error" <- w196
        n72 = Build Array (concatenate)(w214, w196) -> (w219:dbl[])
        n73 = feedback #5() -> (w194:dbl[])  [unwired: 1 in]
        n74 = Build Array (concatenate)(w193, w194) -> (w195:dbl[])
        n75 = Array Size(array=w219) -> (size(s)=w218:i32)
        n76 = Subtract(x=w218, y="Derivative Long History") -> (x-y=w192:i32)
        n77 = Array Subset(array=w195, length=w192) -> (w191:dbl[])  [unwired: 1 in]
        n78 = feedback-in #5(w191) -> ()
        n79 = Subtract(x=w227, y=w226) -> (x-y=w223:dbl)
        n80 = Multiply(x="Derivative Long History", y=0.75) -> (x*y=w201:dbl)
        n81 = Array Subset(array=w219, index=w192) -> (w204:dbl[])  [unwired: 1 in]
        n82 = Array Max & Min(array=w191) -> (max value=w190:dbl, min value=w189:dbl)  [unwired: 2 out]
        n83 = Subtract(x=w190, y=w189) -> (x-y=w188:dbl)
        n84 = Greater?(x=w188, y=0.05) -> (0:w186:bool)
        n85 = In Range and Coerce(upper limit=w224, x=w223, lower limit=w225) -> (coerced(x)=w211:dbl)  [unwired: 1 out]
        n86 = Add(x=w211, y=w216) -> (x+y=w215:dbl)
        n87 = Build Array (concatenate)(w209, w215) -> (w220:dbl[])
        n88 = Array Subset(array=w220, index=w192) -> (w217:dbl[])  [unwired: 1 in]
        n89 = Multiply(x="Kp", y=w196) -> (x*y=w208:dbl)
        "Proportional Term" <- w208
        "Proportional" <- w208
        n90 = Array Size(array=w204) -> (size(s)=w200:i32)
        n91 = call <vilib>:"Linear Fit Coefficients.vi"("Y"=w204, "X"=w217) -> ("slope"=w222:dbl)  [unwired: 3 in, 10 out]
        n92 = Not A Number/Path/Refnum?(number/path/refnum=w222) -> (NaN/Path/Refnum?=w198:bool)
        n93 = Less?(x=w200, y=w201) -> (x < y?=w199:bool)
        n94 = Compound Arithmetic op=OR(w186, w198, w199) -> (w197:bool)
        n95 = Select(t=0.0 ("f"), s=w197, f=w222) -> (s? t:f=w213:dbl)
        n96 = Compound Arithmetic op=MULTIPLY("Ki", w211, w196) -> (w185:dbl)
        n97 = Multiply(x="Kd Long", y=w213) -> (x*y=w207:dbl)
        "Derivative Term" <- w207
        "Derivative Long" <- w207
        n98 = Greater Than 0?(x=w185) -> (x > 0?=w184:bool)
        n99 = Select(t=w183, s=w184, f=w182) -> (s? t:f=w181:bool)
        n100 = Select(t=w177, s=w181, f=w185) -> (s? t:f=w179:dbl)
        n101 = Not A Number/Path/Refnum?(number/path/refnum=w179) -> (NaN/Path/Refnum?=w180:bool)
        n102 = Select(t=w177, s=w180, f=w179) -> (s? t:f=w178:dbl)
      }
      frame #4 {
        n103 = Build Array (concatenate)(w251, string[] ["EnFlo_Lab:Reference:Temperature", "EnFlo_Tunnel:Chiller_Pump:Enable", "EnFlo_Lab:Shut:Down", "EnFlo_Tunnel:Chilled Water:Return", "A_Tunnel:Motor:Enable", "B_Tunnel:Motor:Enable", "D_Tunnel:Motor:Enable", "Aero_Tunnel:Motor:Enable"] ("appended array")) -> (w250:string[])
        n104 = call "Get_Current_Scan_client.vi"("multipleChannels"=w250) -> ("Ch Description Array"=w265:T4[], "Numerical Values"=w248:dbl[])  [unwired: 1 in, 2 out]
        n105 = in-place {
          in-place-border: w262 -> [w283]
          in-place-border: w268 -> [w282]
          in-place-border: w267 -> [w281]
          n106 = in-place-array #6(w265, 1) -> (w285:T4)
          n107 = in-place {
            in-place-border: w283 -> [w289]
            in-place-border: w282 -> [w288]
            in-place-border: w281 -> [w287]
            n108 = in-place-cluster #7(w285) -> ()  [unwired: 1 out]
            n109 = Select(t=w287, s=w289, f=w288) -> (s? t:f=w286:string)
            n110 = in-place-cluster #7("String"=w286) -> (w284:T4)
          }
          n111 = in-place-array #6(w284) -> (w263:T4[])  [unwired: 1 out]
        }
        n112 = Array Subset(array=w248, index=5) -> (w257:dbl[])  [unwired: 1 in]
        n113 = Index Array(array=w248, index #1=0 ("index"), index #2=2 ("index"), index #3=3 ("index"), index #4=4 ("index")) -> (element #1=w239:dbl, element #2=w243:dbl, element #3=w245:dbl, element #4=w232:dbl)
        n114 = Greater Than 0?(x=w235) -> (x > 0?=w234:bool)
        n115 = Greater?(x=w257, y=0.5) -> (0:w256:bool[])
        n116 = Or Array Elements(Boolean array=w256) -> (logical OR=w255:bool)
        n117 = Greater?(x=w243, y=0.5) -> (0:w241:bool)
        n118 = Greater?(x=w245, y=0.5) -> (0:w260:bool)
        n119 = Or(x=w255, y=w254) -> (x .or. y?=w253:bool)
        n120 = feedback-in #8(w241) -> ()
        n121 = feedback #8() -> (w242:bool)  [unwired: 1 in]
        n122 = Compound Arithmetic op=AND(invert w242, w241, w234) -> (w240:bool)
        n123 = case shown="True" w240 {
          tunnel: [w269 w270] -> w230
          tunnel: w239 -> [w269 w271]
          tunnel: w238 -> [_ w279]
          tunnel: w237 -> [_ w278]
          tunnel: w236 -> [_ w277]
          tunnel: w232 -> [_ w276]
          frame False {
          }
          frame True {
            n124 = Search 1D Array(1D array=w279, element=w277) -> (index of element=w280:i32)  [unwired: 1 out]
            n125 = Index Array(array=w278, index=w280) -> (element=w275:dbl)
            n126 = Subtract(x=w276, y=w275) -> (x-y=w274:dbl)
            n127 = Multiply(x=w274, y=0.3) -> (x*y=w272:dbl)
            n128 = Subtract(x=w271, y=w272) -> (x-y=w270:dbl)
          }
        }
        n129 = call "Update_Ch_Discription_server.vi"("Mode"=T3."Append to Global", "Channels to update In"=w263) -> ()  [unwired: 1 in, 1 out]
        n130 = Not A Number/Path/Refnum?(number/path/refnum=w230) -> (NaN/Path/Refnum?=w231:bool)
        n131 = Select(t=0.0, s=w231, f=w230) -> (s? t:f=w228:dbl)
      }
      frame #5 {
        # "Heat input to the lab due to the heating water flowing around is estimated to be about 2.5kW when the water temperature is 70 deg C, and Zero when at 20 deg."
        n132 = Array Size(array=w308) -> (size(s)=w307:i32)
        n133 = Search 1D Array(1D array=w301, element=w299) -> (index of element=w302:i32)  [unwired: 1 out]
        n134 = Index Array(array=w300, index=w302) -> (element=w295:dbl)
        n135 = Subtract(x=w307, y="Derivative Short History") -> (x-y=w312:i32)
        n136 = Array Subset(array=w309, index=w312) -> (w310:dbl[])  [unwired: 1 in]
        n137 = Array Subset(array=w308, index=w312) -> (w311:dbl[])  [unwired: 1 in]
        n138 = Multiply(x=w295, y=0.05) -> (x*y=w298:dbl)
        n139 = Subtract(x=w298, y=1.0) -> (x-y=w293:dbl)
        n140 = call <vilib>:"Linear Fit Coefficients.vi"("Y"=w311, "X"=w310) -> ("slope"=w315:dbl)  [unwired: 3 in, 10 out]
        n141 = Greater Than 0?(x=w293) -> (x > 0?=w294:bool)
        n142 = Not A Number/Path/Refnum?(number/path/refnum=w315) -> (NaN/Path/Refnum?=w313:bool)
        n143 = Select(t=w293, s=w294, f=0.0) -> (s? t:f=→"Heat input to lab from Hot Pipework (kW)":dbl)
        n144 = Select(t=0.0 ("f"), s=w313, f=w315) -> (s? t:f=w305:dbl)
        n145 = Multiply(x="Kd short", y=w305) -> (x*y=w303:dbl)
        "Derivative Short" <- w303
        "EnFlo_Lab Shut Down" <- w290
      }
      frame #6 {
        w336 = 300.0  # Reset Average after Seconds
        w338 = 30  # History length
        w356 = 13  # History length
        w357 = 300.0  # Reset Average after Seconds
        n146 = Max & Min(x=w335, y=w334) -> (max(x,y)=w333:dbl)  [unwired: 1 out]
        n147 = Search 1D Array(1D array=w345, element=w343) -> (index of element=w346:i32)  [unwired: 1 out]
        n148 = Index Array(array=w344, index=w346) -> (element=w337:dbl)
        n149 = Build Array("EnFlo_Tunnel:Chiller_Pump:Running", "Uni:Chilled Water:Temp", "EnFlo_Tunnel:Total Heating:Load (kW)", w322) -> (w318:string[])
        n150 = Search 1D Array(1D array=w345, element=w355) -> (index of element=w359:i32)  [unwired: 1 out]
        n151 = call "Get_Channel_averages.vi"("Desired Ch Names"=w318, "Averaging time (mins)"=w316) -> ("number"=w317:dbl[])  [unwired: 1 in, 2 out]
        n152 = Index Array(array=w344, index=w359) -> (element=w358:dbl)
        n153 = Index Array(array=w317) -> (element #1=w351:dbl, element #2=w326:dbl, element #3=w323:dbl, element #4=w320:dbl)  [unwired: 4 in]
        n154 = feedback #9() -> (w353:dbl[])  [unwired: 1 in]
        n155 = call "Running_Ch_Average.vi"("Shift In"=w353, "History length"=w356, "Reset Average after Seconds"=w357, "New Value"=w358) -> ("Shift Out"=w354:dbl[], "mean"=w349:dbl)  [unwired: 1 in, 1 out]
        n156 = feedback-in #9(w354) -> ()
        n157 = feedback #10() -> (w340:dbl[])  [unwired: 1 in]
        n158 = call "Running_Ch_Average.vi"("Shift In"=w340, "History length"=w338, "Reset Average after Seconds"=w336, "New Value"=w337) -> ("Shift Out"=w339:dbl[], "mean"=w325:dbl)  [unwired: 1 in, 1 out]
        n159 = feedback-in #10(w339) -> ()
        n160 = Greater?(x=w351, y=0.5) -> (0:w332:bool)
        n161 = Greater?(x=w320, y=0.5) -> (0:w319:bool)
        n162 = Select(t=w349, s=w332, f=0.0) -> (s? t:f=w348:dbl)
        n163 = Subtract(x=w333, y=w325) -> (x-y=w342:dbl)
        n164 = Multiply(x=w342, y="Kp Ventilation") -> (x*y=w330:dbl)
        n165 = Greater Than 0?(x=w330) -> (x > 0?=w331:bool)
        n166 = Select(t=w330, s=w331, f=0.0) -> (s? t:f=w329:dbl)
        "Ventilation Cooling limit in kW" <- w329
      }
      frame #7 {
        n167 = Search 1D Array(1D array=w361, element=w373) -> (index of element=w374:i32)  [unwired: 1 out]
        n168 = Search 1D Array(1D array=w361, element=w366) -> (index of element=w371:i32)  [unwired: 1 out]
        n169 = Index Array(array=w360, index=w374) -> (element=w372:dbl)
        n170 = Index Array(array=w360, index=w371) -> (element=w365:dbl)
        n171 = Greater?(x=w365, y=0.5) -> (0:w362:bool)
        n172 = case shown="True" w362 {
          tunnel: w368 -> [w377 w380]
          tunnel: [w375 w378] -> w367
          frame False {
            n173 = Less?(x=w377, y=8.0) -> (x < y?=w375:bool)
          }
          frame True {
            n174 = Greater?(x=w380, y=99.0) -> (0:w378:bool)
          }
        }
        n175 = Compound Arithmetic op=AND(invert w363, w367, w370) -> (w369:bool)
      }
      frame #8 {
        n176 = case shown="False" w389 {
          tunnel: w388 -> [_ w399]
          tunnel: w387 -> [w392 w397]
          tunnel: [w390 w396] -> w386
          tunnel: w385 -> [_ _]
          tunnel: w384 -> [_ _]
          tunnel: w383 -> [_ _]
          tunnel: w382 -> [w393 w395]
          tunnel: w381 -> [w391 _]
          frame False {
            n177 = Subtract(x=w393, y=w391) -> (x-y=w394:dbl)
            n178 = Multiply(x=w394, y=w392) -> (x*y=w390:dbl)
          }
          frame True {
            n179 = Subtract(x=w399, y=w395) -> (x-y=w398:dbl)
            n180 = Multiply(x=w398, y=w397) -> (x*y=w396:dbl)
          }
        }
      }
      frame #9 {
        # "Maximum Heating"
        # "Maximum Heating Integral Term"
        # "Calculate Heat Extraction kW"
        n181 = Multiply(x=w410, y=2.0) -> (x*y=w408:dbl)
        n182 = while {
          shift-right: [w423] -> _
          shift-left: _ -> [w427]
          tunnel: w406 -> [w426]
          tunnel: [w421] -> w405
          stop <- TRUE stop-if-true
          n183 = Build Array (concatenate)(w426, w427) -> (w425:dbl[])
          n184 = Array Subset(array=w425, length=15) -> (w423:dbl[])  [unwired: 1 in]
          n185 = Array Max & Min(array=w423) -> (max value=w421:dbl)  [unwired: 3 out]
        }
        n186 = local read "Heat input to lab from Hot Pipework (kW)"() -> (w414:dbl)
        n187 = Add(x=w412, y=w413) -> (x+y=w402:dbl)
        n188 = Compound Arithmetic op=ADD(w407, w408, w405) -> (w404:dbl)
        n189 = Negate(x=w404) -> (-x=w400:dbl)
        n190 = Greater?(x=w402, y=w400) -> (0:w403:bool)
        n191 = Select(t=w402, s=w403, f=w400) -> (s? t:f=w401:dbl)
        "Integral Term" <- w401
        "integral" <- w401
        n192 = Compound Arithmetic op=ADD(w401, w414, w420, w419, w416) -> (w417:dbl)
        n193 = Not A Number/Path/Refnum?(number/path/refnum=w417) -> (NaN/Path/Refnum?=w418:bool)
        n194 = Select(t=0.0, s=w418, f=w417) -> (s? t:f=w415:dbl)
        "Heat Extraction Value in kW" <- w415
      }
      frame #10 {
        # "Controlling the Lab Fan Heaters"
        n195 = Greater?(x=w452, y=50.0) -> (0:w444:bool)
        n196 = Subtract(x=w451, y=w450) -> (x-y=w447:dbl)
        n197 = Compound Arithmetic op=AND(invert w439, w444, invert "Don't Use Fan Heaters") -> (w443:bool)
        n198 = Add(x=w437, y=w438) -> (x+y=w432:dbl)
        n199 = Greater?(x=w441, y=0.5) -> (0:w440:bool)
        n200 = case shown="False" w443 {
          tunnel: w449 -> [_ w481]
          tunnel: [dbl[] [0.0, 0.0] ("Values") w473] -> w435
          tunnel: w447 -> [_ _]
          tunnel: w446 -> [_ w479]
          tunnel: w445 -> [_ _]
          tunnel: w444 -> [_ _]
          tunnel: w440 -> [_ w465]
          tunnel: w432 -> [_ w472]
          tunnel: w433 -> [_ w467]
          tunnel: w431 -> [_ w466]
          tunnel: w430 -> [_ w459]
          tunnel: [TRUE w456] -> w429
          frame False {
          }
          frame True {
            n201 = Build Array(w481, w479) -> (w461:string[])
            n202 = call "Get_Channel_averages.vi"("Desired Ch Names"=w461, "Averaging time (mins)"=w459) -> ("number"=w460:dbl[])  [unwired: 1 in, 2 out]
            n203 = Index Array(array=w460) -> (element #1=w478:dbl, element #2=w477:dbl)  [unwired: 2 in]
            n204 = Greater Than 0?(x=w478) -> (x > 0?=w480:bool)
            n205 = Greater Than 0?(x=w477) -> (x > 0?=w476:bool)
            n206 = Add(x=w467, y=w467) -> (x+y=w469:dbl)
            n207 = case shown="True" w480 {
              tunnel: w467 -> [w492 w495]
              tunnel: [w492 w493] -> w471
              frame False {
              }
              frame True {
                n208 = Subtract(x=w495, y=0.5) -> (x-y=w493:dbl)
              }
            }
            n209 = Negate(x=w472) -> (-x=w468:dbl)
            n210 = case shown="True" w476 {
              tunnel: w469 -> [w488 w491]
              tunnel: [w488 w489] -> w470
              frame False {
              }
              frame True {
                n211 = Subtract(x=w491, y=0.5) -> (x-y=w489:dbl)
              }
            }
            n212 = case shown="True" w465 {
              tunnel: w468 -> [_ w487]
              tunnel: w467 -> [_ w486]
              tunnel: w466 -> [_ w485]
              tunnel: [TRUE w483] -> w464
              frame False {
              }
              frame True {
                n213 = Add(x=w486, y=w485) -> (x+y=w484:dbl)
                n214 = Greater?(x=w487, y=w484) -> (0:w483:bool)
              }
            }
            n215 = Greater?(x=w468, y=w471) -> (0:w458:bool)
            n216 = Greater?(x=w468, y=w470) -> (0:w457:bool)
            n217 = Select(t=w457, s=w464, f=FALSE) -> (s? t:f=w463:bool)
            n218 = Build Array(w458, w463) -> (w475:bool[])
            n219 = And(x=w458, y=w457) -> (x .and. y?=w456:bool)
            n220 = Boolean To (0,1)(Boolean=w475) -> (0, 1=w474:i16[])
            n221 = To Double Precision Float(number=w474) -> (double precision float=w473:dbl[])
          }
        }
        n222 = Build Array(w449, w446) -> (w448:string[])
        n223 = Add Array Elements(numeric array=w435) -> (sum=w436:dbl)
        n224 = Multiply(x=w436, y=w433) -> (x*y=w434:dbl)
      }
      frame #11 {
        # "Calculate Exit Heater Dem Power %"
        n225 = case shown="False" w506 {
          tunnel: [w515 0.0] -> w505
          tunnel: w504 -> [w515 _]
          tunnel: w502 -> [w514 w520]
          tunnel: w498 -> [_ w519]
          tunnel: w501 -> [_ w518]
          tunnel: [w514 w516] -> w500
          frame False {
          }
          frame True {
            n226 = Add(x=w519, y=w518) -> (x+y=w522:dbl)
            n227 = Negate(x=w522) -> (-x=w521:dbl)
            n228 = Max & Min(x=w520, y=w521) -> (min(x,y)=w516:dbl)  [unwired: 1 out]
          }
        }
        n229 = Less Than 0?(x=w498) -> (x < 0?=w497:bool)
        n230 = Compound Arithmetic op=ADD(w500, w498, w501) -> (w503:dbl)
        n231 = Greater?(x=w512, y=0.5) -> (0:w509:bool)
        n232 = Compound Arithmetic op=AND(w509, w510, w497, invert "Don't Use Exit Heaters") -> (w508:bool)
        n233 = case shown="True" w508 {
          tunnel: w505 -> [_ w536]
          tunnel: [0.0 w527] -> w507
          tunnel: w503 -> [_ w534]
          tunnel: w513 -> [_ w532]
          tunnel: [TRUE w525] -> w499
          frame False {
          }
          frame True {
            w526 = 100.0 ("upper limit")
            n234 = Subtract(x=w534, y=w536) -> (x-y=w535:dbl)
            n235 = Negate(x=w535) -> (-x=w528:dbl)
            n236 = Divide(x=100.0, y=w532) -> (x/y=w531:dbl)
            n237 = Multiply(x=w528, y=w531) -> (x*y=w530:dbl)
            n238 = In Range and Coerce(upper limit=w526, x=w530, lower limit=0.0) -> (coerced(x)=w527:dbl)  [unwired: 1 out]
            n239 = Equal?(x=w526, y=w527) -> (x = y?=w525:bool)
          }
        }
        "Exit Heater Dem Power %" <- w507
      }
      frame #12 {
        # "Calculation of the Lab Ventilation %"
        n240 = Absolute Value(x=w545) -> (abs(x)=w554:dbl)
        n241 = Greater?(x=w554, y=100.0) -> (0:w555:bool)
        n242 = case shown="False" w555 {
          tunnel: w556 -> [_ _]
          tunnel: w553 -> [_ _]
          tunnel: w552 -> [_ _]
          tunnel: w551 -> [_ _]
          tunnel: [w596 w610] -> w546
          tunnel: w550 -> [w595 _]
          tunnel: w549 -> [w594 _]
          tunnel: w548 -> [_ _]
          tunnel: w547 -> [_ _]
          tunnel: w545 -> [_ w613]
          tunnel: w544 -> [w593 _]
          tunnel: w543 -> [w592 _]
          tunnel: w542 -> [_ _]
          tunnel: w541 -> [w591 _]
          tunnel: w540 -> [w589 _]
          tunnel: w539 -> [w588 _]
          tunnel: w538 -> [w587 _]
          tunnel: [w562 TRUE] -> w537
          frame False {
            w582 = 4.5 ("y")
            w590 = 0.0  # Offset
            # "Don't run window ventilation when too cold outside and in working hours and chilled water is available."
            # "Outside air cold and in working hours"
            n243 = Subtract(x=w593, y=w591) -> (x-y=w570:dbl)
            n244 = Build Array("EnFlo_Lab:Volcano Cooler:Fan Power (%)") -> (w565:string[])
            n245 = Greater?(x=w570, y=8.0) -> (0:w566:bool)
            n246 = call "Get_Channel_averages.vi"("Desired Ch Names"=w565, "Averaging time (mins)"=w587) -> ("number"=w564:dbl[])  [unwired: 1 in, 2 out]
            n247 = call "Control value mapping.vi"("Control In%"=w592, "Demand Out%"=dbl[] [60.0, 100.0], "Demand In%"=dbl[] [15.0, 20.0] ("Demand Out%")) -> ("Control Out%"=w576:dbl)
            n248 = Greater?(x=w570, y=w582) -> (0:w583:bool)
            n249 = Index Array(array=w564) -> (element=w572:dbl)  [unwired: 1 in]
            n250 = case shown="False" w583 {
              tunnel: w570 -> [w606 _]
              tunnel: w582 -> [w599 _]
              tunnel: w590 -> [w605 _]
              tunnel: [w602 1.0] -> w580
              frame False {
                n251 = Subtract(x=w606, y=w605) -> (x-y=w604:dbl)
                n252 = Divide(x=w604, y=w599) -> (x/y=w601:dbl)
                n253 = Greater Than 0?(x=w601) -> (x > 0?=w603:bool)
                n254 = Select(t=w601, s=w603, f=0.0) -> (s? t:f=w602:dbl)
              }
              frame True {
              }
            }
            n255 = Build Array(w576, w572, 60.0 ("f")) -> (w574:dbl[])
            n256 = Less?(x=w592, y=14.0) -> (x < y?=w567:bool)
            n257 = Array Max & Min(array=w574) -> (max value=w573:dbl)  [unwired: 3 out]
            n258 = Divide(x=w594, y=w595) -> (x/y=w581:dbl)
            n259 = Compound Arithmetic op=AND(w567, w588, w566) -> (w563:bool)
            n260 = Multiply(x=w581, y=100.0) -> (x*y=w560:dbl)
            n261 = Multiply(x=w580, y=w589) -> (x*y=w579:dbl)
            n262 = Multiply(x=w573, y=w579) -> (x*y=w561:dbl)
            n263 = In Range and Coerce(upper limit=w561, x=w560, lower limit=0.0) -> (coerced(x)=w558:dbl)  [unwired: 1 out]
            n264 = Equal?(x=w561, y=w558) -> (x = y?=w559:bool)
            n265 = case shown="True" w563 {
              tunnel: [w597 TRUE] -> w562
              tunnel: w559 -> [w597 _]
              frame False {
              }
              frame True {
              }
            }
            n266 = Select(t=0.0, s=w563, f=w558) -> (s? t:f=w596:dbl)
          }
          frame True {
            n267 = Greater Than 0?(x=w613) -> (x > 0?=w612:bool)
            n268 = Select(t="Manual Ventilation %", s=w612, f=0.0 ("Ventilation %")) -> (s? t:f=w610:dbl)
          }
        }
      }
      frame #13 {
        w640 = "EnFlo_Tunnel:Ozone:Control  mA" ("Desired Ch to Read")
        n269 = Build Array(w640, "EnFlo_Tunnel Metadata:Ozone:Setpoint(ppb)", "EnFlo_Tunnel:Ozone_Generators:Enable", "D_Tunnel:Motor:Enable") -> (w616:string[])
        n270 = call "Get_Channel_averages.vi"("Desired Ch Names"=w616, "Averaging time (mins)"=w614) -> ("number"=w615:dbl[])  [unwired: 1 in, 2 out]
        n271 = Index Array(array=w615) -> (element #1=w638:dbl, element #2=w639:dbl, element #3=w635:dbl, element #4=w621:dbl)  [unwired: 4 in]
        n272 = Greater?(x=w635, y=0.5) -> (0:w632:bool)
        n273 = Greater?(x=w639, y=1.0) -> (0:w633:bool)
        n274 = And(x=w633, y=w632) -> (x .and. y?=w631:bool)
        n275 = case shown="True" w631 {
          tunnel: w639 -> [_ w684]
          tunnel: w638 -> [_ w657]
          tunnel: [4.0 ("Plot O3 Generator Control %") w664] -> w637
          tunnel: [w645 w652] -> w626
          tunnel: w630 -> [w646 w654]
          tunnel: w621 -> [w649 _]
          frame False {
            n276 = Greater?(x=w649, y=0.5) -> (0:w648:bool)
            n277 = Select(t=0.0, s=w648, f=w646) -> (s? t:f=w645:dbl)
          }
          frame True {
            w658 = 16.0 ("y")
            w659 = 4.0 ("y")
            w668 = 16.0 ("y")
            w666 = 4.0 ("y")
            w674 = dbl[] [1.0, 1.6]  # Demand Out%
            w675 = dbl[] [30.0, 60.0]  # Demand In%
            # "Ozone Setpoint"
            n278 = Subtract(x=w657, y=w659) -> (x-y=w663:dbl)
            n279 = Divide(x=w663, y=w658) -> (x/y=w662:dbl)
            n280 = Build Array("EnFlo_Tunnel:Ozone:(ppb)" ("Desired Ch to Read"), "EnFlo_Lab:SouthWest Window Fan:Power(%)") -> (w683:string[])
            n281 = call "Get_Channel_averages.vi"("Desired Ch Names"=w683, "Averaging time (mins)"="Ozone Averaging time (mins)") -> ("number"=w681:dbl[])  [unwired: 1 in, 2 out]
            n282 = Index Array(array=w681) -> (element #1=w680:dbl, element #2=w672:dbl)  [unwired: 2 in]
            n283 = call "Control value mapping.vi"("Control In%"=w672, "Demand Out%"=w674, "Demand In%"=w675) -> ("Control Out%"=w656:dbl)
            n284 = Divide(x=w662, y=w656) -> (x/y=w661:dbl)
            n285 = Multiply(x=w661, y=w658) -> (x*y=w660:dbl)
            n286 = Add(x=w659, y=w660) -> (x+y=w655:dbl)
            n287 = call "AdjustO3_170926.vi"("O3 Generator Control"="O3 Generator Control", "Control \nO3"=w680, "Target (ppb)"=w684, "Control in"=w655, "Ambient\nO3"=0.0 ("Ambient\nO3"), "O3 ON"=TRUE) -> ("Control out"=w665:dbl)  [unwired: 8 in, 1 out]
            n288 = Subtract(x=w665, y=w666) -> (x-y=w671:dbl)
            n289 = Divide(x=w671, y=w668) -> (x/y=w670:dbl)
            n290 = Multiply(x=w670, y=w656) -> (x*y=w669:dbl)
            n291 = Multiply(x=w669, y=w668) -> (x*y=w667:dbl)
            n292 = Add(x=w666, y=w667) -> (x+y=w664:dbl)
            n293 = Max & Min(x="Lab Ventilation % during Ozone Exp", y=w654) -> (max(x,y)=w652:dbl)  [unwired: 1 out]
          }
        }
        n294 = Build Array(w640) -> (w642:string[])
        n295 = Build Array(w637) -> (w643:dbl[])
        n296 = Or(x=w618, y="Don't Use Ventilation") -> (x .or. y?=w619:bool)
        n297 = call "ASYNC_Adam_server.vi"("Values"=w643, "Channel Names"=w642) -> ()  [unwired: 1 in, 3 out]
        n298 = Select(t=0.0, s=w619, f=w626) -> (s? t:f=w624:dbl)
        n299 = Divide(x=w624, y=100.0) -> (x/y=w628:dbl)
        n300 = Multiply(x=w629, y=w628) -> (x*y=w617:dbl)
        "Ventilation Cooling (kW)" <- w617
        n301 = call "Lab Ventilation.vi"("Paint Spraying by South West Fan"="Paint Spraying by South West Fan", "Ventilation %"=w624) -> ()  [unwired: 1 out]
      }
      frame #14 {
        # "Max allowable %"
        # "Calculation of the Volcano Power"
        n302 = case shown="False" w698 {
          tunnel: w696 -> [_ w706]
          tunnel: [65.0 ("y") w710] -> w686
          tunnel: [1.0 ("f") w705] -> w685
          frame False {
          }
          frame True {
            w708 = dbl[] [0.0, 1.0]  # Demand Out%
            w707 = dbl[] [15.0, 50.0]  # Demand In%
            w712 = 100.0 ("y")
            n303 = Multiply(x=0.005, y=w706) -> (x*y=w716:dbl)
            n304 = Add(x=0.5, y=w716) -> (x+y=w714:dbl)
            n305 = call "Control value mapping.vi"("Control In%"=w706, "Demand Out%"=w708, "Demand In%"=w707) -> ("Control Out%"=w705:dbl)
            n306 = Multiply(x=w714, y=w712) -> (x*y=w711:dbl)
            n307 = In Range and Coerce(upper limit=w712, x=w711, lower limit=0.0) -> (coerced(x)=w710:dbl)  [unwired: 1 out]
          }
        }
        n308 = Or(x=w690, y=w691) -> (x .or. y?=w694:bool)
        n309 = Compound Arithmetic op=AND(invert w687, invert w693, w694) -> (w692:bool)
        n310 = case shown="True" w692 {
          tunnel: w697 -> [_ w728]
          tunnel: [w718 w739] -> w689
          tunnel: w699 -> [_ w738]
          tunnel: w700 -> [_ w737]
          tunnel: w702 -> [_ w736]
          tunnel: w701 -> [_ w735]
          tunnel: [w718 w734] -> w695
          tunnel: [TRUE w727] -> w688
          tunnel: w686 -> [_ w726]
          tunnel: w685 -> [_ w724]
          frame False {
            w718 = 0.0 ("Control Out%")
          }
          frame True {
            # "Max Heat Ex"
            # "Req Heat Extraction"
            n311 = Subtract(x=w738, y=w737) -> (x-y=w725:dbl)
            n312 = Multiply(x=w725, y=w724) -> (x*y=w721:dbl)
            n313 = Subtract(x=w736, y=w735) -> (x-y=w732:dbl)
            n314 = Divide(x=w732, y=12.0) -> (x/y=w730:dbl)
            n315 = Multiply(x=w730, y=w728) -> (x*y=w729:dbl)
            n316 = Greater?(x=w732, y=2.0) -> (0:w723:bool)
            n317 = Greater?(x=w721, y=1.0) -> (0:w719:bool)
            n318 = And(x=w723, y=w719) -> (x .and. y?=w722:bool)
            n319 = case shown="True" w722 {
              selector: w722 -> [w740 _]
              tunnel: w721 -> [_ w748]
              tunnel: w729 -> [_ w744]
              tunnel: [w742 w743] -> w739
              tunnel: [w742 w747] -> w734
              tunnel: [w741 w746] -> w727
              tunnel: w726 -> [_ w745]
              frame False {
                w742 = 0.0 ("Control Out%")
                n320 = Not(x=w740) -> (.not. x?=w741:bool)
              }
              frame True {
                w750 = 100.0 ("y")
                n321 = Divide(x=w748, y=w744) -> (x/y=w753:dbl)
                n322 = Multiply(x=w753, y=w750) -> (x*y=w752:dbl)
                n323 = In Range and Coerce(upper limit=w745, x=w752, lower limit=0.0) -> (coerced(x)=w743:dbl)  [unwired: 1 out]
                n324 = Equal?(x=w745, y=w743) -> (x = y?=w746:bool)
                n325 = Divide(x=w743, y=w750) -> (x/y=w749:dbl)
                n326 = Multiply(x=w744, y=w749) -> (x*y=w747:dbl)
              }
            }
          }
        }
        "Volcano Cooling (kW)" <- w695
      }
      frame #15 {
        # "Calculation of Demanded Exit Duct Temperature"
        n327 = Greater Than 0?(x=w758) -> (x > 0?=w759:bool)
        n328 = And(x=w759, y=w757) -> (x .and. y?=w756:bool)
        n329 = Add(x=w774, y=w773) -> (x+y=w771:dbl)
        n330 = case shown="False" w765 {
          tunnel: w772 -> [w777 _]
          tunnel: w771 -> [w776 _]
          tunnel: [w775 w779] -> w766
          tunnel: w764 -> [_ _]
          tunnel: w763 -> [_ _]
          tunnel: w762 -> [_ w778]
          frame False {
            n331 = Subtract(x=w777, y=w776) -> (x-y=w775:dbl)
          }
          frame True {
            n332 = Negate(x=w778) -> (-x=w779:dbl)
          }
        }
        n333 = case shown="True" w756 {
          tunnel: w758 -> [_ w799]
          tunnel: w766 -> [_ w795]
          tunnel: [w794 w798] -> w768
          tunnel: w757 -> [_ w797]
          tunnel: [w794 w795] -> w760
          frame False {
            w794 = 0.0
          }
          frame True {
            n334 = case shown="False" w797 {
              tunnel: w795 -> [w807 _]
              tunnel: [w804 TRUE] -> w796
              frame False {
                n335 = Absolute Value(x=w807) -> (abs(x)=w806:dbl)
                n336 = Greater?(x=w806, y=0.5) -> (0:w804:bool)
              }
              frame True {
              }
            }
            n337 = case shown="True" w796 {
              tunnel: w799 -> [_ w803]
              tunnel: [0.0 w802] -> w798
              tunnel: w795 -> [_ w801]
              frame False {
              }
              frame True {
                n338 = Divide(x=w801, y=w803) -> (x/y=w802:dbl)
              }
            }
          }
        }
        "Reduction in air temp from ambient" <- w768
        "Back End Chiller Cooling (kW)" <- w760
        n339 = Equal To 0?(x=w768) -> (x = 0?=w770:bool)
        n340 = case shown="True" w770 {
          tunnel: w769 -> [w782 _]
          tunnel: w768 -> [w781 _]
          tunnel: [w780 w789] -> w767
          tunnel: w761 -> [_ w788]
          tunnel: w755 -> [_ w787]
          tunnel: w754 -> [_ w784]
          frame False {
            n341 = Subtract(x=w782, y=w781) -> (x-y=w780:dbl)
          }
          frame True {
            n342 = Greater?(x=w787, y=50.0) -> (0:w785:bool)
            n343 = Or(x=w785, y=w784) -> (x .or. y?=w783:bool)
            n344 = case shown="False" w783 {
              tunnel: [w792 w793] -> w789
              tunnel: w788 -> [w791 w793]
              frame False {
                n345 = Add(x=w791, y=1.0) -> (x+y=w792:dbl)
              }
              frame True {
              }
            }
          }
        }
        "EnFlo_Tunnel:Exit Duct:Dem Temp" <- w767
      }
      frame #16 {
        n346 = Greater Than 0?(x=w819) -> (x > 0?=w818:bool)
        n347 = Build Array (concatenate)(string[] ["EnFlo_Lab:Volcano Cooler:Fan Power (%)", "EnFlo_Lab:Volcano Cooler:Valve", "EnFlo_Lab:Ventilation Cooling:Available", "EnFlo_Lab:Ventilation Cooling:Used", "EnFlo Lab:Heat:Extraction", "EnFlo_Tunnel:Exit Duct:Dem Temp", "EnFlo_Tunnel:Power:Exit_Heaters", "EnFlo_Tunnel:Chiller Cooling:Load (kW)"] ("appended array"), w811) -> (w810:string[])
        n348 = Add(x=w816, y=w815) -> (x+y=w814:dbl)
        n349 = Select(t=w814, s=w818, f=0.0) -> (s? t:f=w813:dbl)
        n350 = Compound Arithmetic op=ADD(w821, w813) -> (w820:dbl)
        n351 = local read "Integral Term"() -> (w809:dbl)
        n352 = Greater Than 0?(x=w826) -> (x > 0?=w834:bool)
        n353 = Select(t=1.0, s=w834, f=0.0) -> (s? t:f=w831:dbl)
        n354 = Build Array (concatenate)(w823, w810) -> (w822:string[])
        n355 = Build Array (concatenate)(w824, w826, w831, w830, w829, w827, w825, w828, w820, w809) -> (w835:dbl[])
        n356 = call "ASYNC_Adam_server.vi"("Values"=w835, "Channel Names"=w822) -> ()  [unwired: 1 in, 3 out]
      }
      frame #17 {
        # "Are we currently on the maximum cooling rate?"
        n357 = Greater Than 0?(x=w840) -> (x > 0?=w841:bool)
        n358 = Compound Arithmetic op=AND(w836, w839, invert w837) -> (w838:bool)
        n359 = case shown="True" w838 {
          tunnel: w851 -> [_ w864]
          tunnel: w850 -> [_ w863]
          tunnel: w849 -> [_ w862]
          tunnel: w848 -> [_ w860]
          tunnel: w847 -> [_ w858]
          tunnel: w846 -> [_ w857]
          tunnel: [TRUE w854] -> w842
          frame False {
          }
          frame True {
            n360 = Search 1D Array(1D array=w864, element=w863) -> (index of element=w865:i32)  [unwired: 1 out]
            n361 = Index Array(array=w862, index=w865) -> (element=w861:dbl)
            n362 = Max & Min(x=w860, y=w861) -> (max(x,y)=w859:dbl)  [unwired: 1 out]
            n363 = Greater?(x=w857, y=96.0) -> (0:w855:bool)
            n364 = Less?(x=w859, y=w858) -> (x < y?=w853:bool)
            n365 = Compound Arithmetic op=AND(w853, w855) -> (w854:bool)
          }
        }
        "Back End Chiller Cooling Max" <- w842
        n366 = Compound Arithmetic op=AND(w845, w844, w842, w841) -> (w843:bool)
        "At Maximum Cooling" <- w843
      }
      frame #18 {
        # "Are we currently on the maximum heating rate?"
        n367 = And(x=w874, y=w873) -> (x .and. y?=w872:bool)
        n368 = case shown="False" w872 {
          tunnel: w875 -> [_ w883]
          tunnel: [TRUE w881] -> w878
          tunnel: [FALSE w881] -> w868
          frame False {
          }
          frame True {
            n369 = Greater?(x=w883, y=98.0) -> (0:w881:bool)
          }
        }
        "Back End Chiller Heating Max" <- w868
        n370 = Less Than 0?(x=w866) -> (x < 0?=w867:bool)
        n371 = Compound Arithmetic op=AND(w877, w876, w878, w867) -> (w869:bool)
        "At Maximum Heating" <- w869
        "Vent Max" <- w871
        "Volcano Max" <- w870
        "Fan Heater Max" <- w876
        "Exit Heaters Max" <- w877
      }
    }
  }
